vi "对非本VI中控件属性操作.vi"() -> ()   [LabVIEW 2018]
uses:
  <vilib>/Utility/error.llb/DialogType.ctl
  <vilib>/Utility/miscctls.llb/LVPointTypeDef.ctl
  <vilib>/Utility/file.llb/Read Delimited Spreadsheet (string).vi
  <vilib>/Utility/file.llb/Write Delimited Spreadsheet (string).vi
panel:
  in  "下拉列表":T1 items=["Digital"]
  in  "界面控件":T2 {"下拉列表" items=["Digital"]}
  in  "选项卡控件":enum32{"基本设置", "控件外观设置", "创建控件"}(tab)
  in  "获取控件名称":bool
  in  "重定原点":bool
  in  "获取控件引用":bool
  in  "流量控件设置":bool
  in  "电流控件设置":bool
  in  "温度控件设置":bool
  in  "压力压差控件设置":bool
  in  "创建数量":u16
  in  "创建T控件":bool
  in  "停止":bool
  out "Error Report":string
  out "Dynamic Threads Array":string[](array[string])
  out "Current State":string
  in  "OK":bool
  in  "Exit Program":bool
  in  "Load Dynamic VI":bool
  in  "Close Dynamic VI":bool
  in  "Load Engine VI":bool
  in  "Close Engine VI":bool
  in  "Load Reentrant VI":bool
  out "数值":i32
  in  "颜色盒 2":u32(colorbox)
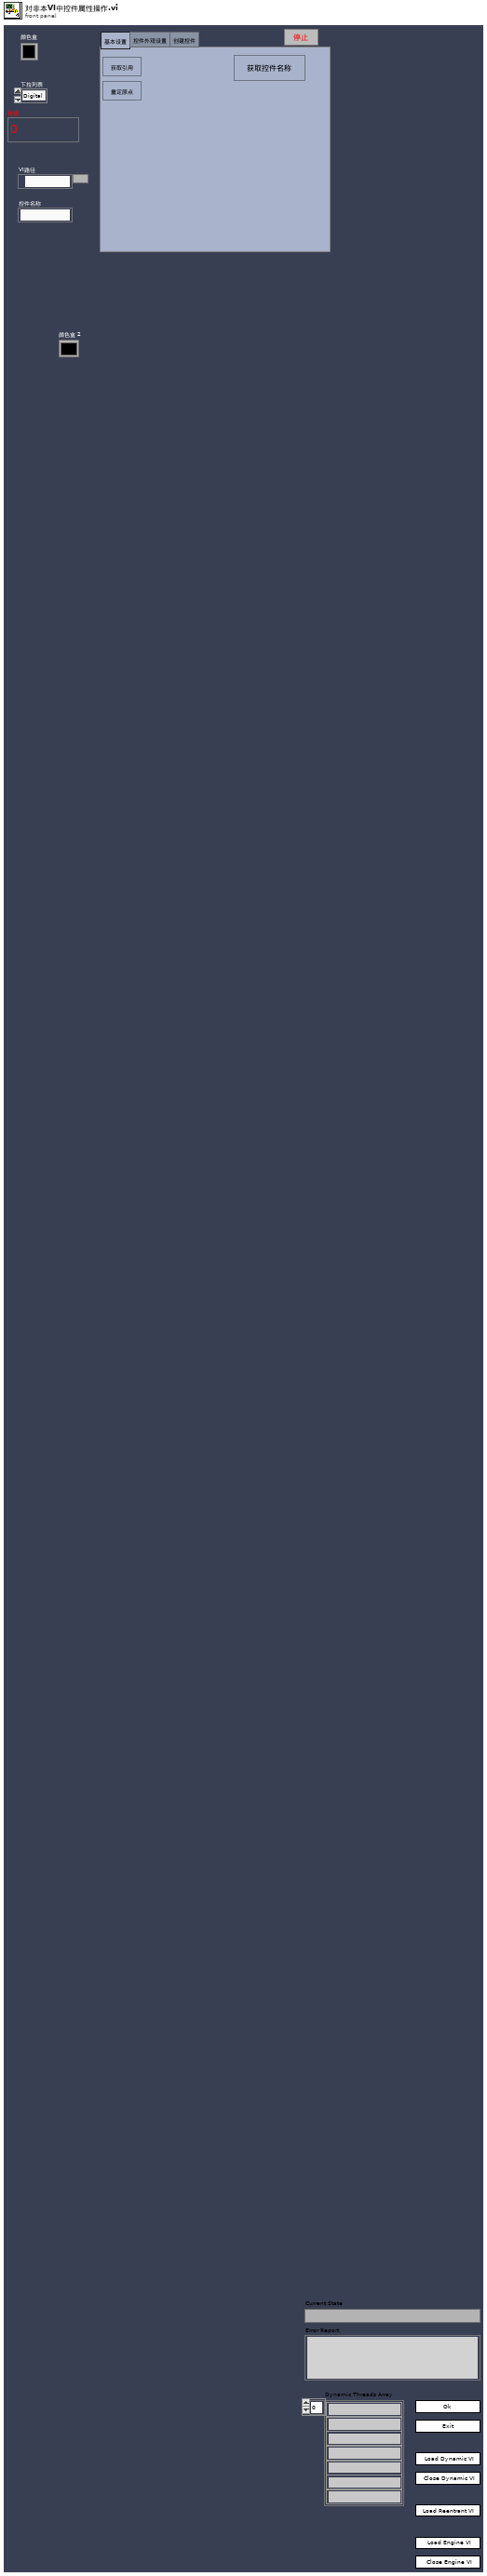
[diagram p1: front panel]
types:
  T1 = typedef "类名.ctl" = u16
  T2 = cluster{"颜色盒":u32, "下拉列表":T1, "VI路径":path, "控件名称":string}
  T3 = typedef "LVPointTypeDef.ctl" = cluster{"Horizontal":i16, "Vertical":i16}
  T4 = typedef "LVBoundsTypeDef.ctl" = cluster{"Width":u32, "Height":u32}
  T5 = typedef "LVFontTypeDef.ctl" = cluster{"Font Name":string, "Size":u16, "Bold":bool, "Italic":bool, "Underline":bool, "Strikeout":bool, "Color":u32}
  T6 = typedef "DynamicThreads.ctl" = cluster{"ReOriginVI":path}
  T7 = cluster{"Error":errorcluster, "Exit":bool, "All Ref":cluster{"VIRef":refnum<vi>, "CtlRef":refnum<vi>, "界面控件Ref":refnum<vi>}, "System Path":cluster{"Data":path}, "Dynamic VI Path":cluster{"Thread Path":path}, "Reentrant VI Path":cluster{"Reentrant Thread Path":path, "Reentrant VI Count":u32}, "Engine Path":cluster{"Engine Path":path}, "Main VI":cluster{"Main Name":string, "Main Order":string, "Main Data":variant}, "Engine":cluster{"Engine Path":path, "Engine Name":string, "Engine Order":string, "Engine Data":variant}, "Thread to Operate":cluster{"Thread VI Path":path, "Invoke Property":cluster{"open front panel? (T)":bool, "Reentrant? (F)":bool, "Insert to Subpanel?(F)":bool, "time out(5s)":dbl}, "Queue Info":cluster{"HighLevel Thread":string, "Thread Q Name":string, "Data":variant}}, "Send Data to Thread":cluster{"Thread to Send":string[], "Order to Send":string[], "Data to Send":variant[]}, "Dynamic Threads Array":string[], "控件排布前面板":cluster{"获取引用":cluster{"获取VI引用句柄":refnum<vi>, "获取Ctl引用句柄":refnum<vi>}, "位置_前":cluster{"位置":T3}, "创建控件":cluster{"创建数量":u16}, "lNameLable":string[]}, "控件排布后面板":cluster{"位置_后":cluster{"位置":T3}}, "DynamicThreadsPath":T6, "界面控件":cluster{"当前选择路径":path, "控件名称":string, "颜色盒":u32, "名称列表路径":path, "名称列表":string[], "类名":string}}
  T8 = enum32{"Invalid", "Standard", "Closed", "Hidden", "Minimized", "Maximized"}
  T9 = cluster{"open front panel? (T)":bool, "Reentrant? (F)":bool, "Insert to Subpanel?(F)":bool, "time out(5s)":dbl}
  T10 = typedef "DialogType.ctl" = u16
  T11 = cluster{"HighLevel Thread":string, "Thread Q Name":string, "Data":variant}
  T12 = cluster{"颜色盒":bool, "下拉列表":bool, "VI路径":bool, "控件名称":bool}
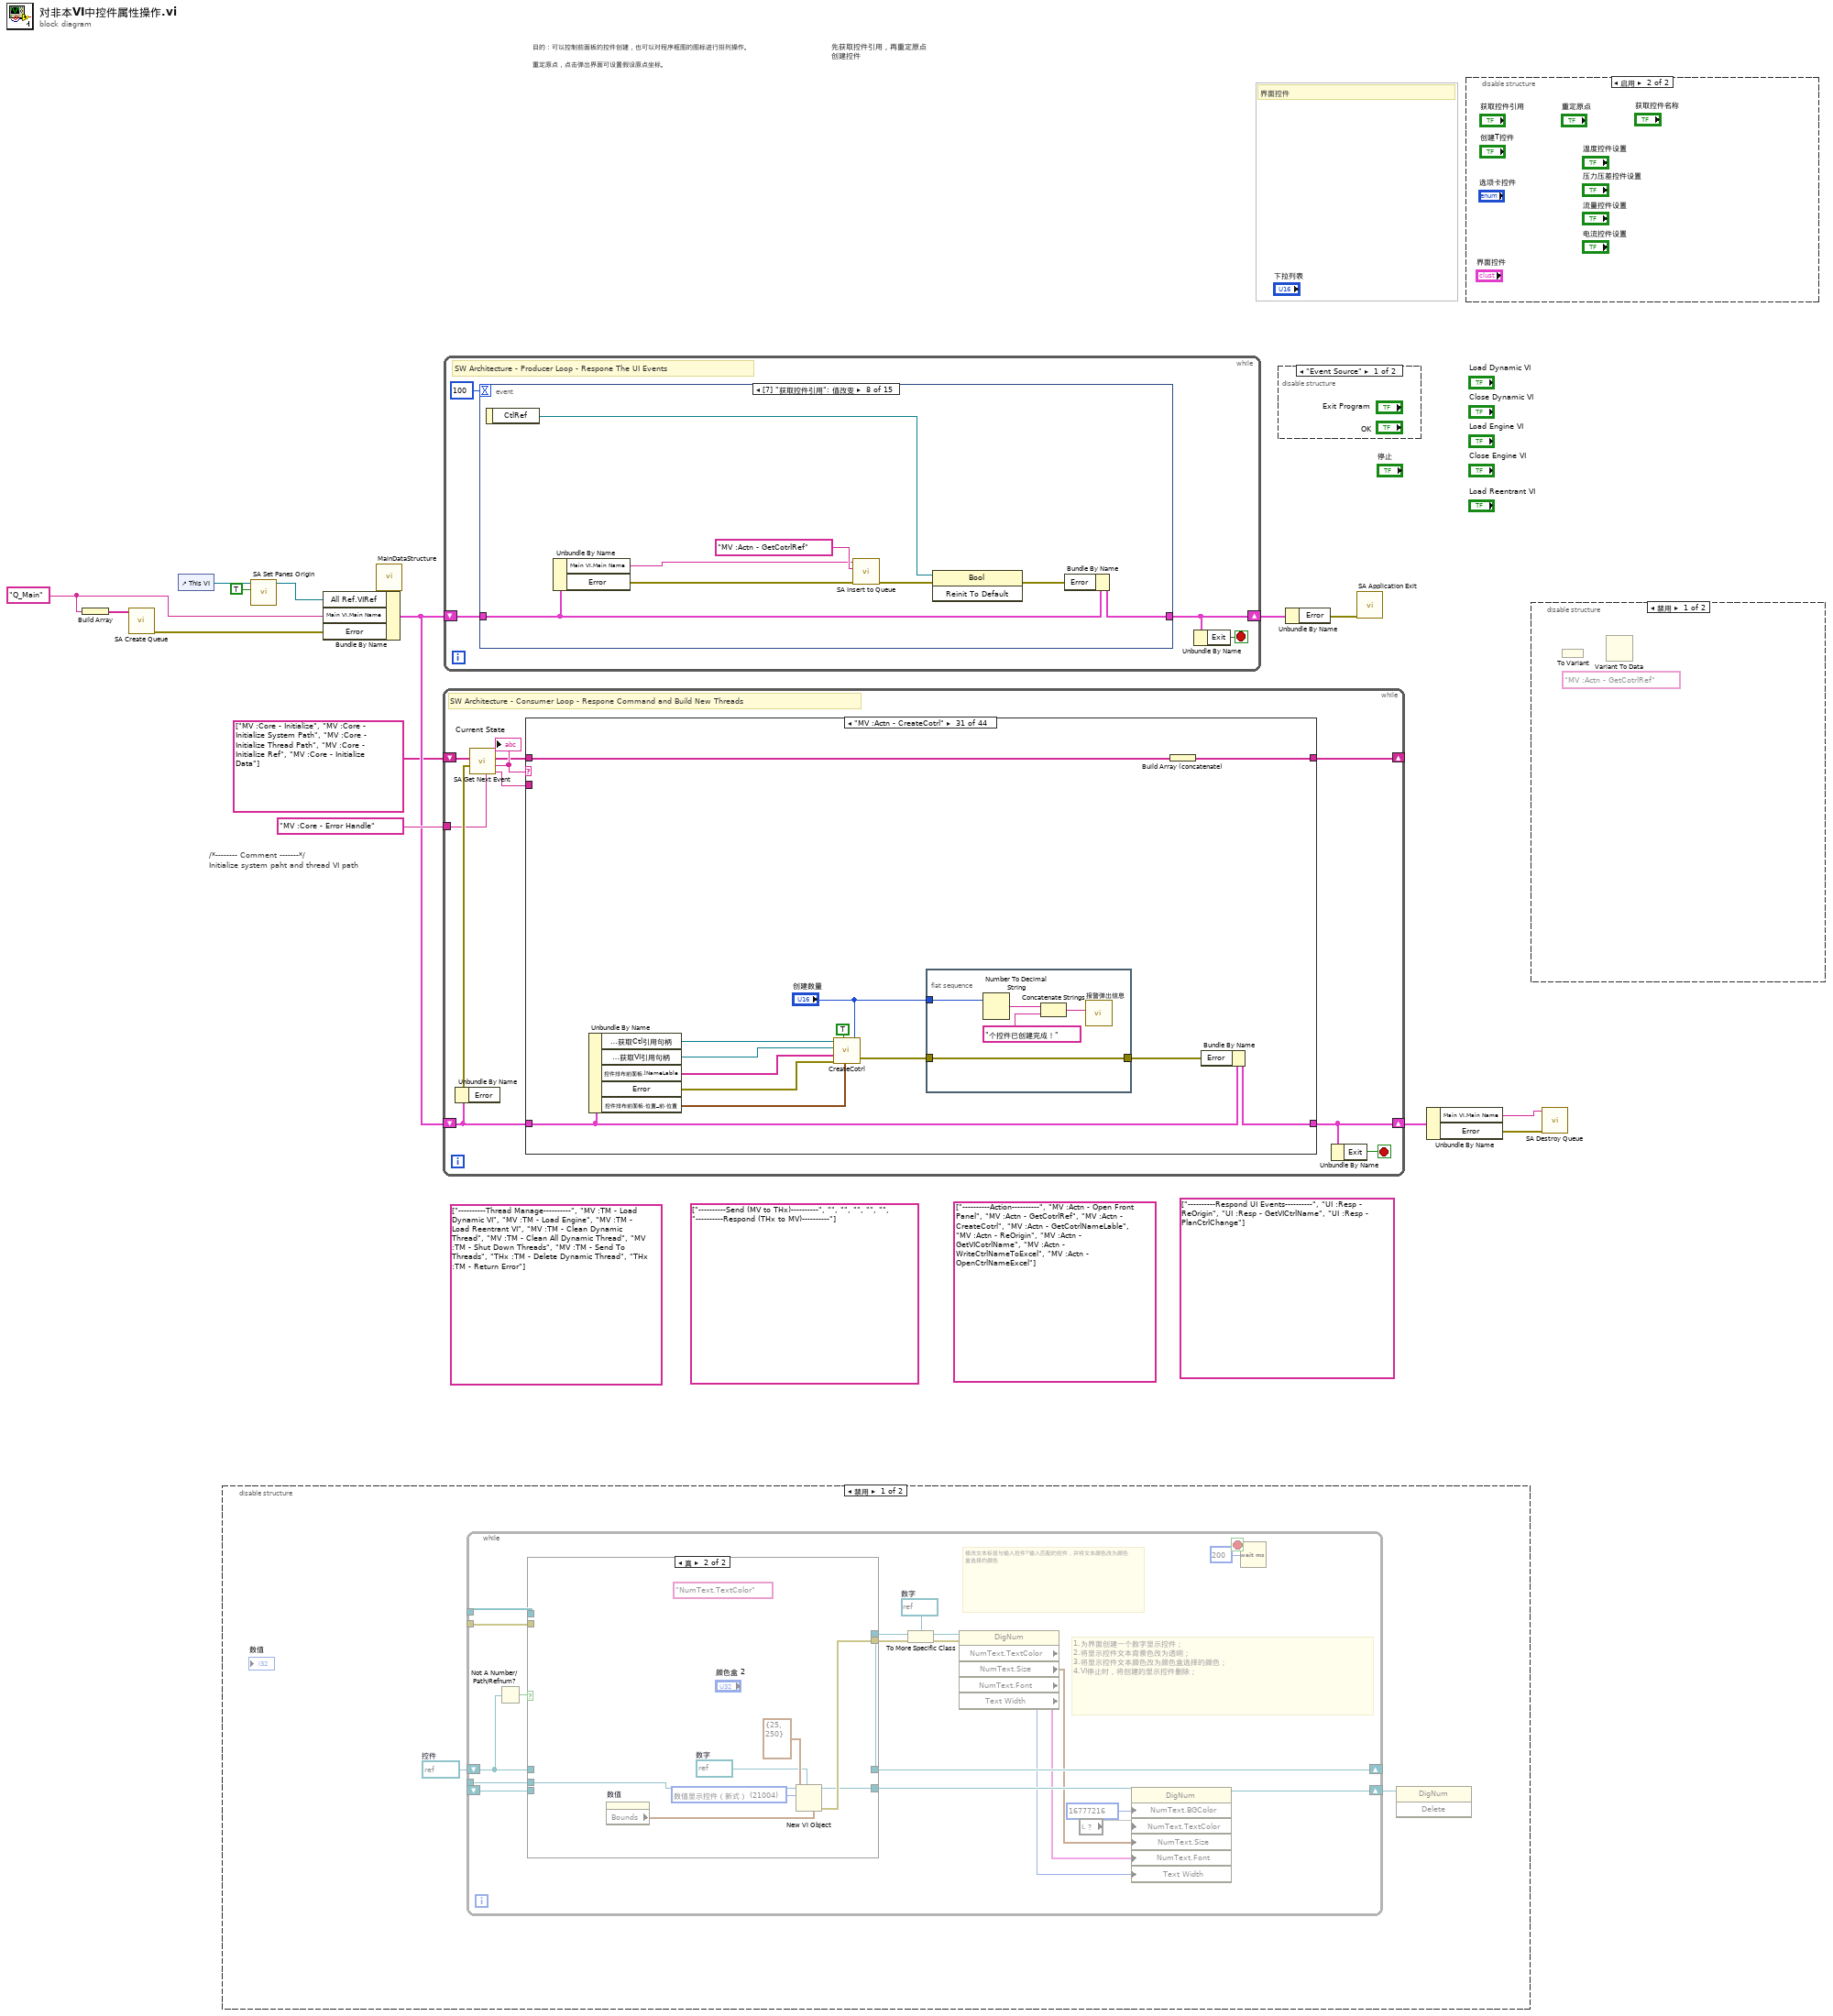
[diagram p0: block diagram]
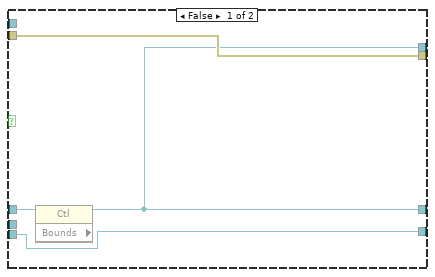
[diagram p4: hidden frame]
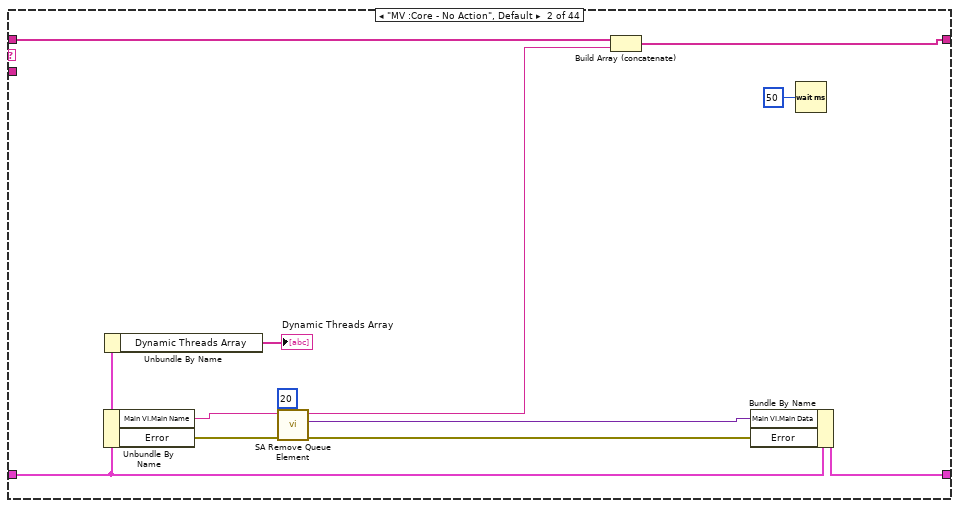
[diagram p8: hidden frame]
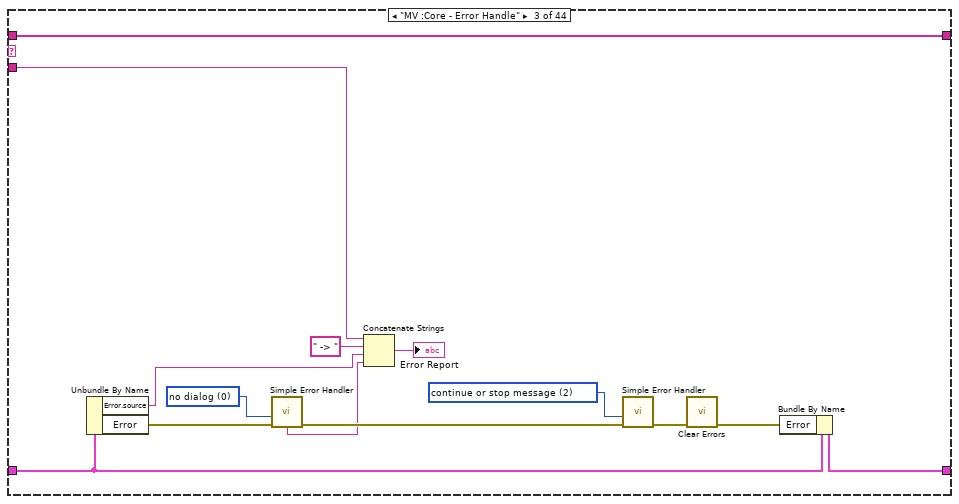
[diagram p9: hidden frame]
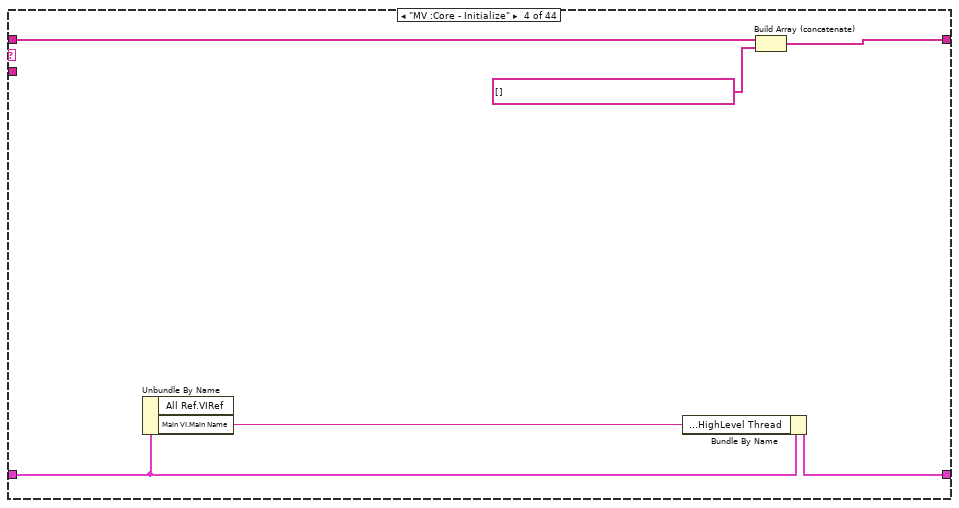
[diagram p10: hidden frame]
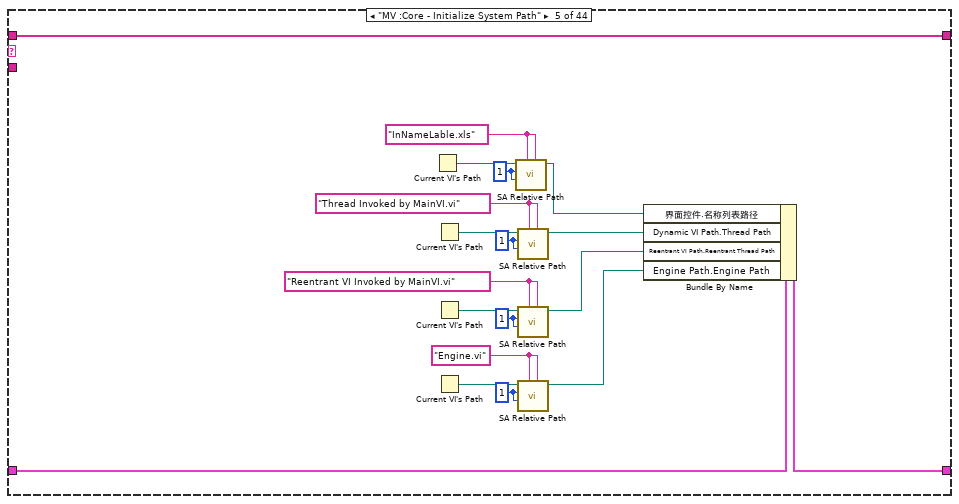
[diagram p11: hidden frame]
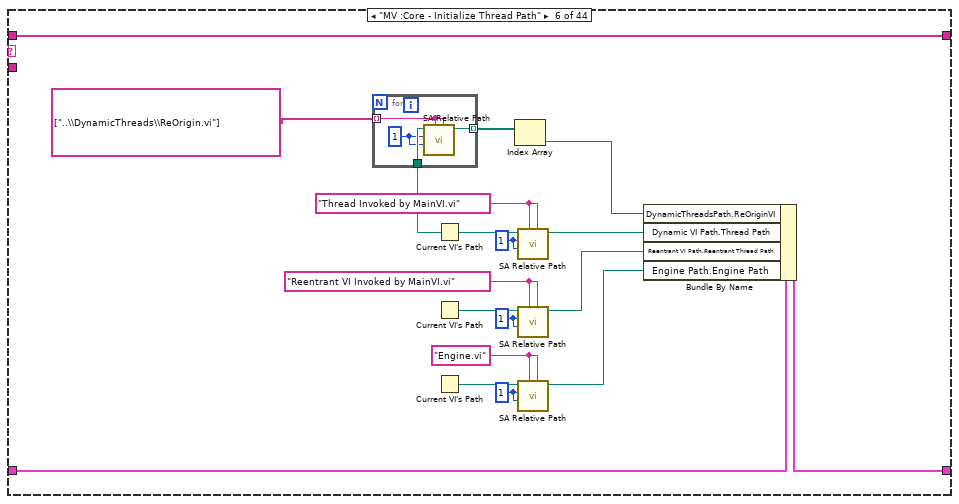
[diagram p12: hidden frame]
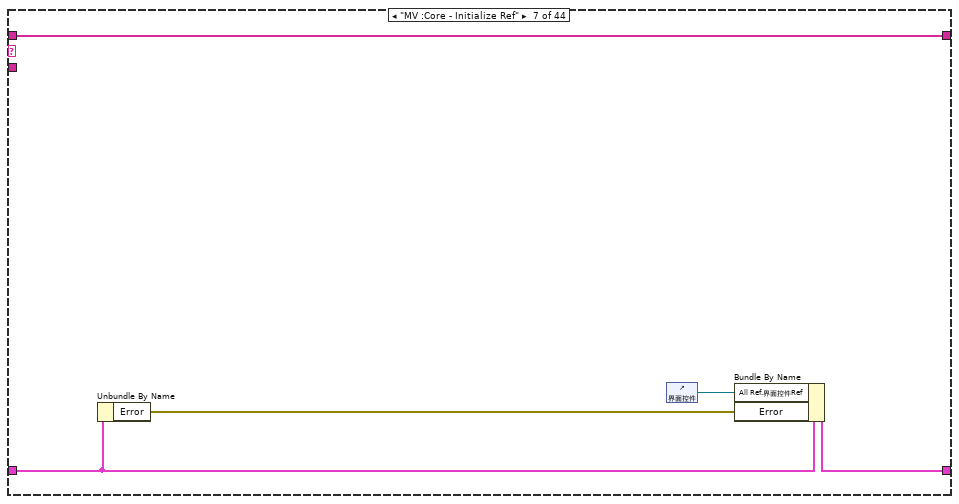
[diagram p13: hidden frame]
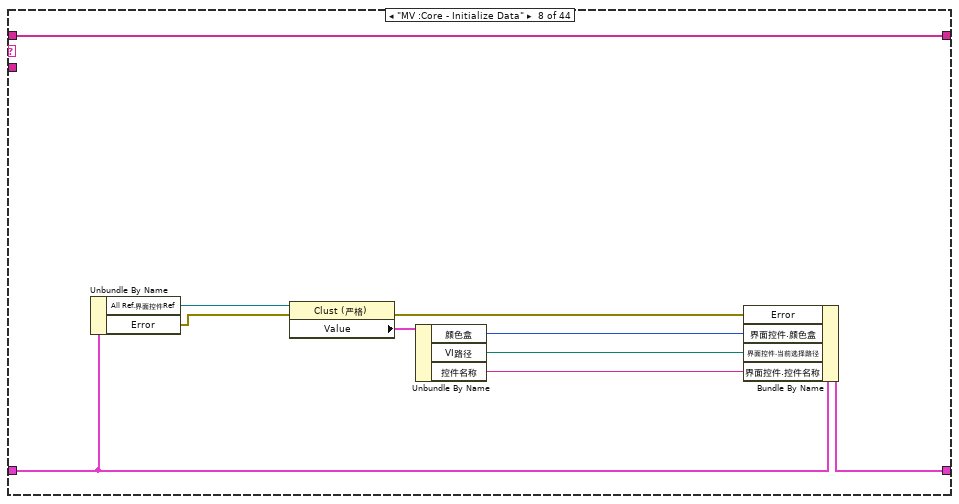
[diagram p14: hidden frame]
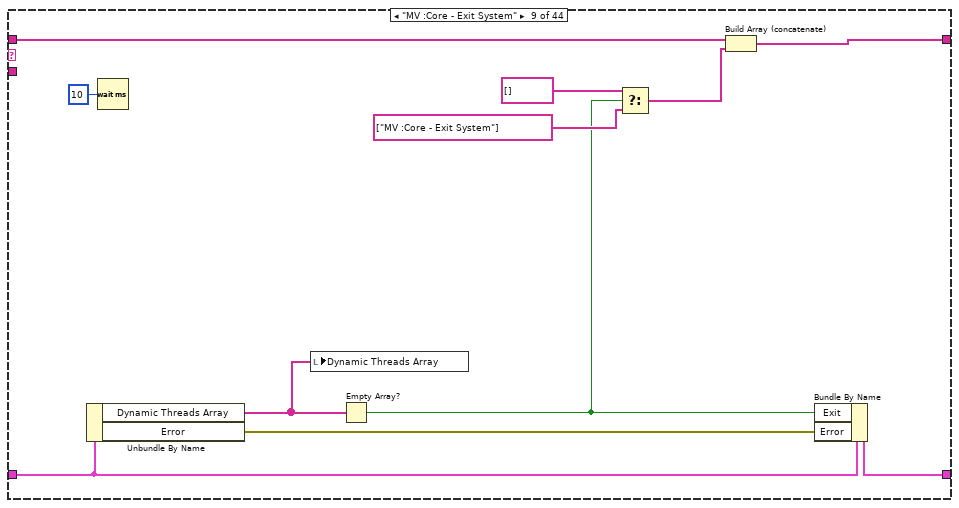
[diagram p15: hidden frame]
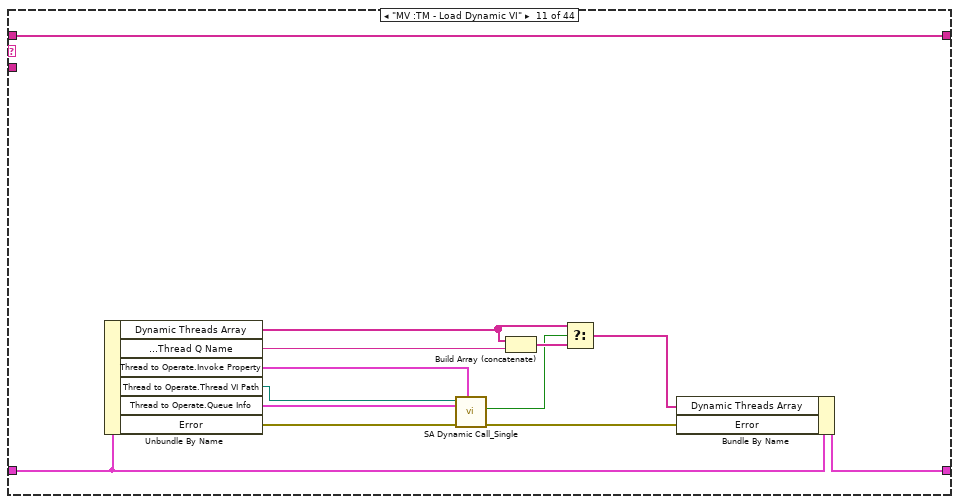
[diagram p17: hidden frame]
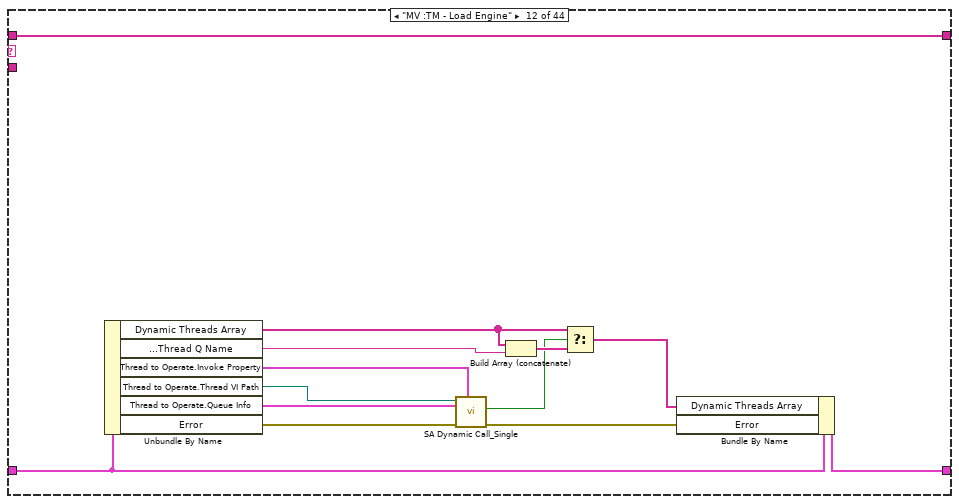
[diagram p18: hidden frame]
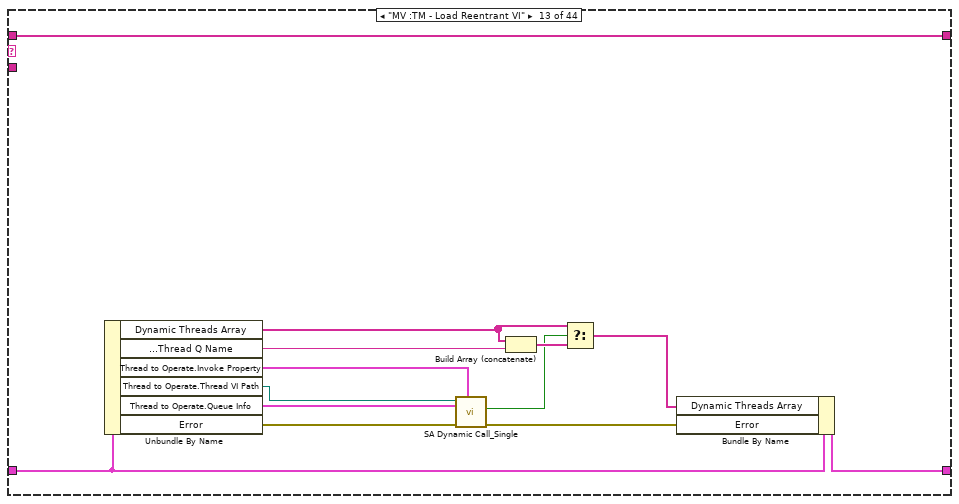
[diagram p19: hidden frame]
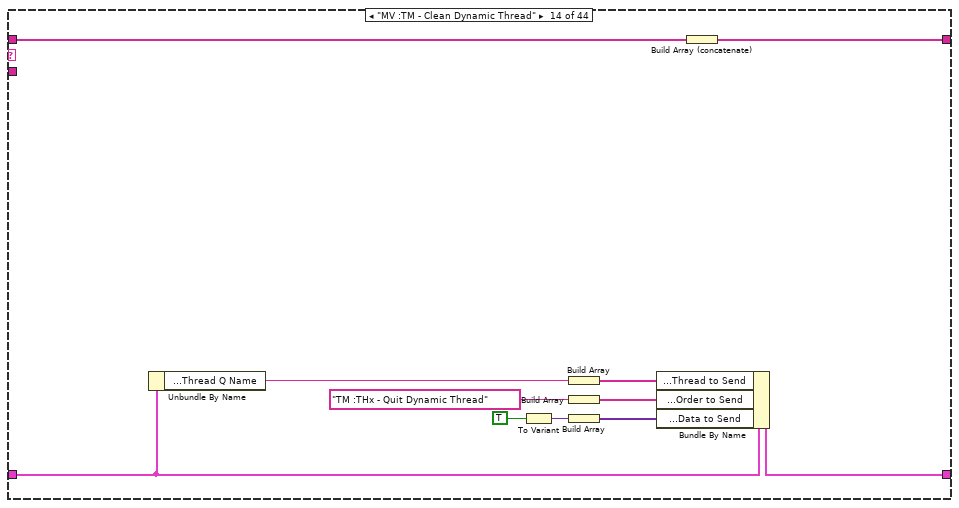
[diagram p20: hidden frame]
diagram:
  (unwired) string[] ["----------Action----------", "MV :Actn - Open Front Panel", "MV :Actn - GetCotrlRef", "MV :Actn - CreateCotrl", "MV :Actn - GetCotrlNameLable", "MV :Actn - ReOrigin", "MV :Actn - GetVICotrlName", "MV :Actn - WriteCtrlNameToExcel", "MV :Actn - OpenCtrlNameExcel"]
  (unwired) string[] ["----------Respond UI Events----------", "UI :Resp - ReOrigin", "UI :Resp - GetVICtrlName", "UI :Resp - PlanCtrlChange"]
  (unwired) string[] ["----------Send (MV to THx)----------", "", "", "", "", "", "----------Respond (THx to MV)----------"]
  (unwired) string[] ["----------Thread Manage----------", "MV :TM - Load Dynamic VI", "MV :TM - Load Engine", "MV :TM - Load Reentrant VI", "MV :TM - Clean Dynamic Thread", "MV :TM - Clean All Dynamic Thread", "MV :TM - Shut Down Threads", "MV :TM - Send To Threads", "THx :TM - Delete Dynamic Thread", "THx :TM - Return Error"]
  w9 = "Q_Main" ("Queue name(unamed)")
  # "界面控件"
  # "目的：可以控制前面板的控件创建，也可以对程序框图的图标进行排列操作。\n\n重定原点，点击弹出界面可设置假设原点坐标。"
  # "先获取控件引用，再重定原点\n创建控件"
  # "/*-------- Comment -------*/\nInitialize system paht and thread VI path"
  n1 = Build Array(w9) -> (w10:string[])
  n2 = call <vilib>:"SA Create Queue.vi"("Queue Name"=w10) -> ("error out"=w6:errorcluster)  [unwired: 10 in]
  n3 = control-ref of="This VI"() -> (w13:refnum<vi>)
  n4 = disable-structure shown="禁用" {
    frame Disabled {
      w18 = refnum<vi> refnum  # 控件
      n5 = while {
        tunnel: _ -> [w38]
        tunnel: _ -> [w39]
        shift-right: [w31] -> _
        shift-left: w18 -> [w29]
        tunnel: [w27] -> w16
        shift-right: [w24] -> w17
        shift-left: _ -> [w22]
        stop <- _ stop-if-true
        w36 = refnum<vi> refnum  # 数字
        # "修改文本标签与输入控件Y输入匹配的控件，并将文本颜色改为颜色盒选择的颜色"
        # "1.为界面创建一个数字显示控件；\n2.将显示控件文本背景色改为透明；\n3.将显示控件文本颜色改为颜色盒选择的颜色；\n4.VI停止时，将创建的显示控件删除；"
        n6 = Not A Number/Path/Refnum?(number/path/refnum=w29) -> (NaN/Path/Refnum?=w30:bool)
        n7 = case shown="真" w30 {
          tunnel: w39 -> [w43 _]
          tunnel: w38 -> [_ _]
          tunnel: [w43 w48] -> w33
          tunnel: [w41 w47] -> w28
          tunnel: [w41 w47] -> w31
          tunnel: w29 -> [w42 _]
          tunnel: w27 -> [_ w46]
          tunnel: [w40 w45] -> w23
          tunnel: w22 -> [w40 _]
          frame False {
            n8 = property class="Ctl" props=["Bounds"](reference=w42) -> (reference out=w41:refnum<vi>)  [unwired: 1 in, 2 out]
          }
          frame True {
            w49 = refnum<vi> refnum  # 数字
            w51 = 21004 items=[".NET容器"=2125, ".NET引用句柄"=3441, "10的幂"=1212, "10的自然对数"=23513, "2的幂"=1223, "2的自然对数"=23514, "ActiveX容器"=2072, "Agitator"=3831, "Array Interface Control"=23777, "Bin#1"=3073, "Bin#2"=21755, "CAN接口（程序框图常量）"=2123, "CAN接口（经典）"=3339, "CAN接口（系统）"=21964, "CAN接口（新式）"=21815, "CAN任务（程序框图常量）"=3471, "CAN任务（经典）"=3470, "CAN任务（系统）"=21963, "CAN任务（新式）"=21789, "CAN通道（程序框图常量）"=2124, "CAN通道（经典）"=3340, "CAN通道（系统）"=21966, "CAN通道（新式）"=21817, "CPU信息"=24130, "DAQmx换算名（程序框图常量）"=2116, "DAQmx换算名（经典）"=3317, "DAQmx换算名（系统）"=21952, "DAQmx换算名（新式）"=21775, "DAQmx接线端（程序框图常量）"=2117, "DAQmx接线端（经典）"=3319, "DAQmx接线端（系统）"=21955, "DAQmx接线端（新式）"=21781, "DAQmx开关（程序框图常量）"=2121, "DAQmx开关（经典）"=3337, "DAQmx开关（系统）"=21953, "DAQmx开关（新式）"=21776, "DAQmx模拟触发器源（程序框图常量）"=2119, "DAQmx模拟触发器源（经典）"=3336, "DAQmx模拟触发器源（系统）"=21951, "DAQmx模拟触发器源（新式）"=21774, "DAQmx全局通道（程序框图常量）"=3430, "DAQmx全局通道（经典）"=3443, "DAQmx全局通道（系统）"=21957, "DAQmx全局通道（新式）"=21770, "DAQmx任务名（程序框图常量）"=3434, "DAQmx任务名（经典）"=3442, "DAQmx任务名（系统）"=21959, "DAQmx任务名（新式）"=21778, "DAQmx设备名（程序框图常量）"=2093, "DAQmx设备名（经典）"=3318, "DAQmx设备名（系统）"=21950, "DAQmx设备名（新式）"=21773, "DAQmx物理通道（程序框图常量）"=2118, "DAQmx物理通道（经典）"=3335, "DAQmx物理通道（系统）"=21954, "DAQmx物理通道（新式）"=21777, "DataSocket引用句柄"=3417, "EOF"=1410, "exp(x)-1"=1222, "e的倒数"=23511, "FieldPoint IO点（程序框图常量）"=3440, "FieldPoint IO点（经典）"=3439, "FieldPoint IO点（新式）"=21784, "FIFO引用句柄"=3474, "For循环"=2002, "FPGA引用句柄至会话句柄转换"=2322, "Furnace"=3829, "GPIB初始化"=1957, "GPIB触发"=1953, "GPIB串行轮询"=1955, "GPIB等待"=1958, "GPIB读取"=1951, "GPIB其他命令"=1956, "GPIB清零"=1954, "GPIB写入"=1950, "GPIB状态"=1959, "IMAQ会话句柄"=3415, "IP地址至字符串转换"=1710, "IVI逻辑名称（程序框图常量）"=3420, "IVI逻辑名称（经典）"=3414, "IVI逻辑名称（新式）"=21736, "IVI删除会话句柄"=8103, "IVI新建会话句柄"=8102, "LabVIEW对象"=3457, "Mac对话组合框"=32514, "MathScript节点"=2357, "MATLAB脚本"=9020, "OLE变体"=3150, "Pi"=23504, "Pi乘以2"=23505, "Pi除以2"=23506, "Pi的倒数"=23507, "Pi的自然对数"=23508, "Python会话引用句柄"=3486, "Python节点"=24205, "RT FIFO创建"=24000, "RT FIFO读取"=24001, "RT FIFO删除"=24003, "RT FIFO写入"=24002, "Simon量表"=32600, "Sinc"=1227, "TCP平化读取"=1718, "TCP平化写入"=1719, "TCP网络连接引用句柄"=3407, "TCP自由读取"=1720, "TCP自由写入"=1721, "TDMS Close"=24113, "TDMS Defragment"=24119, "TDMS Flush"=24117, "TDMS Get Properties"=24115, "TDMS List Contents"=24116, "TDMS Open"=24112, "TDMS Read"=24111, "TDMS Refnum To File ID"=24120, "TDMS Set Properties"=24114, "TDMS Write"=24110, "TDMS Write IP"=24118, "TDMS获取异步读取状态（数据引用）"=2155, "TDMS获取异步写入状态（数据引用）"=2154, "TDMS内存中打开"=2156, "TDMS内存中读取字节"=2158, "TDMS内存中关闭"=2157, "TDMS配置异步读取（数据引用）"=2153, "TDMS配置异步写入（数据引用）"=2152, "TDMS删除数据"=2159, "TDMS文件"=3477, "UDP网络连接引用句柄"=3418, "UTF-8至文本转换"=23067, "VISA GPIB传递IFC"=2318, "VISA GPIB传递控制权"=2317, "VISA GPIB控制ATN"=2316, "VISA GPIB控制REN"=2304, "VISA GPIB命令"=2315, "VISA USB控制输出"=2087, "VISA USB控制输入"=2086, "VISA VXI命令或查询"=2305, "VISA查找资源"=1923, "VISA存数16"=1935, "VISA存数32"=1996, "VISA存数64"=2143, "VISA存数8"=1939, "VISA打开"=2308, "VISA等待事件"=1943, "VISA读取"=1925, "VISA读取STB"=1928, "VISA读取设备并写入文件"=2313, "VISA读取文件并写入设备"=2314, "VISA放弃事件"=1941, "VISA关闭"=1922, "VISA解锁"=1994, "VISA禁用事件"=1940, "VISA内存分配"=1997, "VISA内存分配Ex"=2146, "VISA内存释放"=1998, "VISA启用事件"=1942, "VISA清空I/O缓冲区"=2302, "VISA取数16"=1934, "VISA取数32"=1995, "VISA取数64"=2142, "VISA取数8"=1938, "VISA取消触发映射"=2312, "VISA取消地址映射"=1933, "VISA设备清零"=1927, "VISA设置I/O缓冲区大小"=2301, "VISA输出16"=1931, "VISA输出32"=1945, "VISA输出64"=2141, "VISA输出8"=1937, "VISA输入16"=1930, "VISA输入32"=1944, "VISA输入64"=2140, "VISA输入8"=1936, "VISA锁"=1993, "VISA写入"=1926, "VISA引用句柄至会话句柄转换"=2300, "VISA映射触发"=2311, "VISA映射地址"=1932, "VISA置触发有效"=1929, "VISA置效用信号有效"=2310, "VISA置中断信号有效"=2309, "VISA转出16"=1949, "VISA转出32"=1992, "VISA转出64"=2145, "VISA转出8"=1947, "VISA转入16"=1948, "VISA转入32"=1991, "VISA转入64"=2144, "VISA转入8"=1946, "VISA转移"=2303, "VISA状态说明"=1924, "VISA资源名称"=3421, "VISA资源名称（经典）"=3409, "VISA资源名称（新式）"=21737, "VI服务器引用"=2091, "VI库"=1425, "VI引用句柄"=3422, "While循环#1"=2003, "While循环#2"=2352, "XY图（经典）"=3500, "XY图（新式）"=21716, "X的Y次根"=23062, "X的幂"=1213, "阿伏加德罗常数(1/mol)"=23520, "按2的幂缩放"=1074, "按名称解除捆绑"=2058, "按名称捆绑"=2057, "按索引获取控件值"=24204, "按索引设置控件值"=24203, "八进制数？"=1129, "八进制字符串至数值转换"=1186, "包矩阵"=23001, "包括定点溢出状态"=5564, "保留运行类"=8018, "比特包至数组"=3135, "闭包结构"=2372, "变量类说明符常量"=2106, "变量名称常量"=3478, "变体"=3310, "变体至平化字符串转换"=8203, "变体至数据转换"=8003, "标签（系统）"=21961, "标签（新式）"=21960, "标识符属性下拉列表"=2063, "表达式节点"=2201, "表格（经典）"=21796, "表格（系统）"=21797, "表格（新式）"=21790, "并行轮询"=1969, "并行轮询配置"=1970, "波形图（经典）"=3504, "波形图（新式）"=21703, "波形图表"=21010, "波形图表（经典）"=3501, "波形图表（新式）"=21717, "不等于0？"=1116, "不等于？"=1105, "布尔数组至数值转换"=1815, "布尔值至(0,1)转换"=1167, "步进数值控件（系统）"=21900, "彩色矩形（断开？）"=3625, "菜单下拉列表（经典）"=3018, "菜单下拉列表（新式）"=21600, "菜单引用句柄"=3413, "测试SRQ"=1986, "层叠式顺序结构"=2000, "插入菜单项"=9003, "插入式控件"=21820, "查找请求设备"=1966, "查找通道探针"=9155, "查找侦听器"=1965, "拆分按钮"=21020, "拆分路径"=1420, "拆分数字"=1170, "拆分信号"=2351, "拆分一维数组"=1908, "产生前面板活动"=1329, "产生事件发生"=1700, "产生用户定义Trace事件"=2250, "产生用户事件"=2074, "敞口槽（经典）"=3070, "敞口槽（新式）"=21751, "敞口罐（平面，经典）"=21752, "敞口罐（阴影，经典）"=3074, "乘"=1052, "乘（带错误接线端）"=3917, "程序框图禁用结构"=2054, "抽取一维数组"=2046, "初始化数组"=2053, "除"=1053, "除（带错误接线端）"=3918, "触发"=1988, "触发设备列表"=1989, "传递控制权"=1968, "传送器"=3827, "传统DAQ通道（程序框图常量）"=2085, "传统DAQ通道（经典）"=3320, "传统DAQ通道（新式）"=21733, "串行轮询所有设备"=1960, "创建TCP侦听器"=1717, "创建波形"=2066, "创建簇数组"=2047, "创建红外线侦听器"=9140, "创建矩阵"=8500, "创建蓝牙侦听器"=9151, "创建流"=23796, "创建路径"=1419, "创建数组"=2041, "创建网络流读取方端点"=23811, "创建网络流端点"=23793, "创建网络流写入方端点"=23810, "创建唯一网络流读取方端点"=23807, "创建唯一网络流端点"=23795, "创建唯一网络流写入方端点"=23806, "创建文件夹"=8055, "创建用户事件"=2073, "垂直分隔栏"=21860, "垂直分隔栏（经典）"=21862, "垂直分隔栏（系统）"=21864, "垂直管道（平面）"=3816, "垂直管道（阴影）"=3716, "垂直滚动条"=21111, "垂直滑动杆（系统）"=21903, "垂直滑动杆开关（经典）"=3115, "垂直滑动杆开关（新式）"=21741, "垂直进度条（系统）"=21909, "垂直进度条（新式）"=21104, "垂直开关"=3109, "垂直刻度条"=21107, "垂直平滑盒"=3634, "垂直翘板开关"=21740, "垂直梯度矩形"=32503, "垂直梯度椭圆"=32501, "垂直梯度圆角矩形"=32506, "垂直填充滑动杆（经典）"=3009, "垂直填充滑动杆（新式）"=21014, "垂直摇杆开关（经典）"=3111, "垂直摇杆开关（新式）"=21005, "垂直直线"=3822, "垂直指针滑动杆（经典）"=3007, "垂直指针滑动杆（系统）"=21901, "垂直指针滑动杆（新式）"=21017, "从JSON还原"=24202, "从XML还原"=8401, "从流中读取单个元素"=23797, "从流中读取多个元素"=23803, "从之前设备中读取数据"=1972, "从字符串还原"=1165, "簇（经典）"=3400, "簇（新式）"=21607, "簇常量"=2071, "簇至数组转换"=1169, "错误下拉列表常量"=2039, "打开/创建/替换数据记录文件"=8054, "打开/创建/替换文件"=8050, "打开DataSocket"=1084, "打开Python会话"=24206, "打开TCP连接"=1715, "打开UDP"=1723, "打开UDP多点传送"=1727, "打开VI对象引用"=8013, "打开VI引用"=8010, "打开变量连接"=23779, "打开并验证变量连接"=23790, "打开动态比特文件引用"=5691, "打开红外线连接"=9142, "打开蓝牙连接"=9153, "打开设备"=1430, "打开文件"=1403, "打开应用程序引用"=8012, "打开自动化"=8000, "大于0？"=1117, "大于？"=1110, "大于等于0？"=1114, "大于等于？"=1103, "带边框颜色盒（经典）"=3008, "带边框颜色盒（新式）"=21019, "带标签方形按钮"=3123, "带标签矩形按钮"=3124, "带标签椭圆形按钮"=3125, "带标签圆形按钮"=3122, "带箭头线（粗）"=3631, "带箭头线（细）"=3628, "带进位的右移位"=1607, "带进位的左移位"=1606, "带阴影的椭圆"=32509, "带阴影的圆角矩形"=32508, "代码接口节点"=2050, "单按钮对话框"=1340, "单位转换"=2059, "单选按钮（经典）"=22003, "单选按钮（系统）"=3133, "单选按钮（系统） 1"=22002, "单选按钮（新式）"=22001, "弹出菜单下拉列表"=3017, "当前VI菜单栏"=9000, "当前VI路径"=1426, "当前进程ID"=24131, "倒数"=1059, "等待(ms)"=1302, "等待GPIB RQS"=1952, "等待SRQ"=1990, "等待TCP侦听器"=1712, "等待带通知器历史的多个通知"=9132, "等待带通知器历史的通知"=9131, "等待多个通知"=9106, "等待红外线侦听器"=9143, "等待活动"=1722, "等待蓝牙侦听器"=9147, "等待前面板活动"=1328, "等待事件发生"=1701, "等待通知"=9105, "等待下一个整数倍毫秒"=1327, "等于0？"=1113, "等于？"=1102, "底数为10的对数"=1210, "底数为2的对数"=1225, "底数为X的对数"=1224, "电子表格字符串至数组转换"=1539, "调用父方法"=2354, "调用节点"=3900, "调用库函数节点"=2062, "调用链"=1999, "调整矩阵大小"=8508, "定点溢出？"=5565, "定点转换为整型"=5566, "定时顺序"=5573, "定时循环"=5570, "动态FPGA接口转换"=5690, "读取DataSocket"=1086, "读取TCP数据"=1716, "读取UDP数据"=1724, "读取变量"=23781, "读取变量（超时方式）"=23786, "读取二进制文件"=8051, "读取红外线数据"=9145, "读取蓝牙数据"=9149, "读取设备"=1432, "读取数据记录文件"=8069, "读取文本文件"=8070, "读取文件"=1407, "读取状态"=1973, "队列引用句柄"=3424, "队列最前端插入元素"=9129, "对话框垂直滚动条"=21906, "对话框数值#1"=2100, "对话框数值#2"=3006, "对话框水平滚动条"=21905, "对话框字符串"=2110, "多段管道"=23780, "多列列表框（经典）"=21799, "多列列表框（系统）"=21798, "多列列表框（新式）"=21791, "多速率结构"=2199, "二维数组转置"=1902, "二维图片"=3508, "发动机（平面）"=3820, "发动机（阴影）"=3720, "发送"=1977, "发送IFC"=1980, "发送LLO"=1982, "发送命令"=1978, "发送设置"=1983, "发送数据"=1979, "发送通知"=9104, "发送至设备列表"=1981, "反馈节点"=2353, "反双曲余割"=23056, "反双曲余切"=23058, "反双曲余弦"=1218, "反双曲正割"=23057, "反双曲正切"=1219, "反双曲正弦"=1217, "反余割"=23050, "反余切"=23052, "反余弦"=1207, "反正割"=23051, "反正切"=1208, "反正切（2个输入）"=1228, "反正弦"=1206, "反转一维数组"=1900, "反转字符串"=1537, "方形按钮"=3101, "方形单选按钮"=3107, "方形灯"=3105, "方形开关按钮"=3119, "方形开关按钮（性能分析）"=3113, "方形指示灯（经典）"=3121, "方形指示灯（新式）"=21013, "访问权限"=1412, "非"=1064, "非法共享变量"=23527, "非法路径常量"=23524, "非法数字/路径/引用句柄？"=1128, "非法引用句柄常量"=23526, "分叉"=2194, "分解变体"=2404, "分解锁定数据变量引用"=2406, "分数/指数字符串至数值转换"=1187, "符号"=1049, "浮点数等于？"=23064, "复共轭"=1048, "复合运算"=2200, "复数至极坐标转换"=1045, "复数至实部虚部转换"=1044, "复选框（经典）"=3117, "复选框（系统）"=3132, "复选框（新式）"=21924, "复制"=8053, "复制（过时）"=1416, "负无穷大"=23509, "高级TDMS异步读取（数据引用）"=2151, "高级TDMS异步写入（数据引用）"=2150, "格式化日期/时间字符串"=8100, "格式化写入文件"=2083, "格式化写入字符串"=2081, "格式化值"=1512, "公式节点"=2004, "共享变量"=23778, "共享变量常量"=3473, "共享变量控件（经典）"=3472, "共享变量控件（新式）"=21814, "共享变量至字符串转换"=1831, "构造器节点"=3904, "关闭DataSocket"=1085, "关闭Python会话"=24207, "关闭TCP连接"=1713, "关闭UDP"=1726, "关闭变量连接"=23783, "关闭红外线连接"=9144, "关闭蓝牙连接"=9148, "关闭文件"=8052, "关闭文件（已停用 ）"=1405, "关闭引用"=8011, "关闭自动化"=8001, "合并错误"=2147, "合并信号"=2350, "红外线网络连接引用句柄"=3450, "滑动开关"=21011, "缓存级别数量"=24133, "换行符常量"=23501, "回车键常量"=23500, "回调事件引用句柄"=3435, "会话句柄至引用句柄转换"=2307, "混合复选框（系统）"=21333, "混合信号图"=21721, "获取帮助窗口状态"=1354, "获取变体属性"=8205, "获取波形成分"=2067, "获取波形属性"=8208, "获取菜单项信息"=9005, "获取定点分量"=11163, "获取队列引用"=9108, "获取队列状态"=9110, "获取记录数量"=8064, "获取矩阵对角"=8501, "获取矩阵元素"=8502, "获取卷信息"=8067, "获取快捷菜单信息"=9007, "获取权限"=8065, "获取日期/时间（秒）"=1303, "获取日期/时间字符串"=1600, "获取数据记录位置"=8061, "获取所选菜单项"=9001, "获取通知器引用"=9101, "获取通知器状态"=9103, "获取拖放数据"=9154, "获取文件大小"=8063, "获取文件类型和创建者"=8066, "获取文件位置"=8062, "获取子矩阵"=8503, "或"=1062, "或非"=1072, "基本单位转换"=1079, "极坐标至复数转换"=1047, "极坐标至实部虚部转换"=23061, "计算机Epsilon"=23528, "加"=1050, "加1"=1057, "加（带错误接线端）"=3915, "假常量"=2006, "检查结构类型是否匹配"=2416, "检查值"=3833, "简易垂直滑动杆"=3002, "简易数值"=2900, "简易水平滑动杆"=3003, "简易字符串"=2115, "减"=1051, "减1"=1058, "减（带错误接线端）"=3916, "交叉"=2197, "交换器"=3828, "交换向量元素"=1912, "交换值"=2401, "交换字"=1163, "交换字节"=1162, "交织一维数组"=2045, "接收数据"=1974, "截取字符串"=1503, "解除捆绑"=2048, "经典垂直滑动杆"=3004, "经典水平滑动开关"=3114, "经典颜色盒"=3013, "经典颜色梯度"=3022, "静态VI引用"=2084, "竞争结构"=2371, "旧VISA打开"=1921, "局部变量"=2061, "矩形停止按钮"=3128, "矩阵大小"=8507, "矩阵转置"=8509, "拒绝访问"=8057, "句柄存数"=1605, "句柄取数"=1604, "卷信息"=1414, "绝对值"=1054, "开关按钮"=21001, "可打印？"=1124, "空白？"=1125, "空路径常量"=23523, "空数组？"=23063, "空字符串/路径？"=1112, "空字符串常量"=23503, "控件引用句柄"=3419, "控件与仿真循环"=2099, "控制帮助窗口"=1353, "控制在线帮助"=1355, "捆绑"=2049, "蓝牙网络连接引用句柄"=3468, "类说明符常量"=2094, "类型"=2414, "类型必须为簇"=2418, "类型必须为数组"=2417, "类型错误"=2415, "类型和创建者"=1434, "类型专用结构"=2373, "里德伯常数(1/m)"=23521, "连接"=2195, "连接字符串"=2040, "量表（经典）"=3040, "量表（新式）"=21009, "列表框（经典）"=21806, "列表框（系统）"=21805, "列表框（新式）"=21792, "列表框符号下拉列表控件常量"=2038, "列表目录"=1418, "临时目录"=1435, "漏斗#1"=21754, "漏斗#2"=3072, "路径常量"=2009, "路径类型"=1421, "路径至字符串数组转换"=1423, "路径至字符串转换"=1077, "罗列文件夹"=8083, "逻辑移位"=1081, "枚举（经典）"=3023, "枚举（系统）"=3062, "枚举（新式）"=21605, "枚举常量"=2090, "秒至日期/时间转换"=1309, "摩尔气体常数(J/(mol K))"=23522, "默认目录"=1427, "内嵌C节点"=2104, "判定范围并强制转换"=1127, "匹配模式"=1535, "匹配真/假字符串"=1533, "匹配字符串"=1532, "平方"=23059, "平方根"=1060, "平滑的椭圆"=32500, "平滑的圆角矩形"=32505, "平化至JSON"=24201, "平化至XML"=8400, "平化至字符串"=1164, "平化字符串至变体转换"=8202, "平面反向三角形"=3623, "平面方形按钮"=3103, "平面盒"=3602, "平面框"=3608, "平面右向三角形"=3621, "平面圆盒"=3611, "平面圆形"=3605, "平面圆形按钮"=3102, "平面正向三角形"=3622, "平面左向三角形"=3620, "平铺式顺序结构"=2069, "平台平面方形按钮"=3134, "普朗克常数(J/Hz)"=23516, "启用本地模式"=1963, "启用菜单跟踪"=9002, "启用远程模式"=1964, "强度图（经典）"=3510, "强度图（新式）"=21720, "强度图表（经典）"=3509, "强度图表（新式）"=21719, "强制类型转换"=1166, "强制转换至类型"=2402, "翘板开关"=21002, "清除定点溢出状态"=5562, "清空队列"=9114, "清空事件队列"=2135, "请求释放内存"=1610, "区域"=2196, "取负数"=1069, "取消按钮（系统）"=3131, "取消按钮（新式）"=21739, "取消并行轮询配置"=1971, "取消释放变体值引用"=2411, "取消通知"=9107, "取消注册会话句柄"=2320, "取消注册事件"=2076, "全局变量"=2060, "确定按钮（系统）"=3130, "确定按钮（新式）"=21738, "日期/时间至秒转换"=1308, "三维图片"=23776, "扫描变量读取"=23784, "扫描变量写入"=23787, "扫描文件"=2082, "扫描值"=1534, "扫描字符串"=2080, "删除"=8056, "删除（过时）"=1417, "删除变体属性"=8206, "删除波形属性"=8209, "删除菜单项"=9004, "删除定点溢出状态"=5563, "删除数据值引用"=2409, "删除数组元素"=3912, "商与余数"=1056, "上矩形值（轮廓）"=21762, "上矩形值（平面）"=3702, "上矩形值（阴影）"=3802, "上凸反向三角形"=3615, "上凸盒（经典）"=3600, "上凸盒（新式）"=3637, "上凸框"=3606, "上凸右向三角形"=3613, "上凸圆盒"=3609, "上凸圆形"=3603, "上凸正向三角形"=3614, "上凸左向三角形"=3612, "设备控制/状态"=1433, "设备清零"=1961, "设备清零列表"=1962, "设备引用句柄"=3405, "设置RWLS"=1984, "设置变体属性"=8204, "设置波形属性"=8207, "设置菜单项信息"=9006, "设置超时"=1985, "设置记录数量"=8075, "设置矩阵对角"=8504, "设置矩阵元素"=8505, "设置句柄大小"=1603, "设置权限"=8076, "设置事件发生"=1702, "设置数据记录位置"=8072, "设置文件大小"=8074, "设置文件类型和创建者"=8077, "设置文件位置"=8073, "设置子矩阵"=8506, "生成地址"=1967, "十进制数？"=1119, "十进制数字符串至数值转换"=1184, "十六进制数？"=1123, "十六进制数字符串至数值转换"=1185, "时间标识（程序框图常量）"=2068, "时间标识输入控件（经典）"=5555, "时间标识输入控件（系统）"=21967, "时间标识输入控件（新式）"=21913, "时间标识显示控件（经典）"=5556, "时间标识显示控件（新式）"=21914, "时间计数器"=1300, "实部虚部至复数转换"=1046, "实部虚部至极坐标转换"=23060, "事件发生引用句柄"=3406, "事件回调注册"=2078, "事件结构"=2052, "事件数据节点"=2102, "释放变体值引用"=2410, "释放队列引用"=9109, "释放通知器引用"=9102, "首次调用？"=1083, "属性节点"=1920, "树形控件（经典）"=21819, "树形控件（系统）"=21794, "树形控件（新式）"=21793, "数据缓冲区大小"=24132, "数据记录文件引用句柄"=3402, "数据值引用"=3476, "数据值引用常量"=24134, "数值常量"=2005, "数值控件（经典）"=3000, "数值控件（系统）"=21919, "数值控件（新式）"=21003, "数值显示控件（经典）"=3001, "数值显示控件（新式）"=21004, "数值至八进制字符串转换"=1182, "数值至布尔数组转换"=1814, "数值至工程字符串转换"=1183, "数值至十进制数字符串转换"=1180, "数值至十六进制字符串转换"=1181, "数值至小数字符串转换"=1506, "数值至指数字符串转换"=1505, "数字波形图（经典）"=3511, "数字波形图（新式）"=21718, "数字数据（经典）"=3210, "数字数据（新式）"=21216, "数组（程序框图常量）"=2070, "数组（经典）"=3300, "数组（新式）"=21608, "数组插入"=3911, "数组大小"=1809, "数组内存信息"=2412, "数组元素或操作"=1910, "数组元素相乘"=1904, "数组元素相加"=1903, "数组元素与操作"=1911, "数组至比特包"=3136, "数组至簇转换"=1168, "数组至电子表格字符串转换"=1540, "数组子集"=2044, "数组最大值与最小值"=1907, "刷新流"=23808, "刷新文件"=8059, "刷新文件（过时）"=1406, "双按钮对话框"=1341, "双曲余割"=23053, "双曲余切"=23055, "双曲余弦"=1215, "双曲正割"=23054, "双曲正切"=1216, "双曲正弦"=1214, "水平按钮框"=3636, "水平分隔栏"=21861, "水平分隔栏（经典）"=21863, "水平分隔栏（系统）"=21865, "水平管道（平面）"=3810, "水平管道（阴影）"=3710, "水平罐"=3071, "水平滚动条"=21110, "水平滑动杆（经典）"=3010, "水平滑动杆（系统）"=21904, "水平进度条（系统）"=21910, "水平进度条（新式）"=21102, "水平开关"=3108, "水平刻度条"=21106, "水平平滑盒"=3633, "水平梯度矩形"=32504, "水平梯度椭圆"=32502, "水平梯度圆角矩形"=32507, "水平填充滑动杆（经典）"=3012, "水平填充滑动杆（新式）"=21100, "水平线"=3821, "水平摇杆开关（经典）"=3110, "水平摇杆开关（新式）"=21700, "水平指针滑动杆（经典）"=3011, "水平指针滑动杆（系统）"=21902, "水平指针滑动杆（新式）"=21101, "搜索"=1409, "搜索/拆分字符串"=1538, "搜索变量容器"=23802, "搜索红外线"=9141, "搜索蓝牙设备"=9152, "搜索替换字符串"=3914, "搜索一维数组"=1901, "随机数(0-1)"=1070, "索引数组"=2042, "索引与捆绑簇数组"=2056, "索引字符串数组"=1531, "锁定范围"=1411, "替换数组子集"=3910, "替换子字符串"=3913, "添加真/假字符串"=1511, "条件结构"=2001, "条件禁用结构"=2064, "停止"=1350, "停止按钮"=21230, "通过引用调用"=3901, "通过引用调用MathScript"=3906, "通知器引用句柄"=3423, "同或"=1073, "图片下拉列表（经典）"=3015, "图片下拉列表（系统）"=21925, "图片下拉列表（新式）"=21602, "退出LabVIEW"=1352, "尾数与指数"=1150, "未组合的矩阵"=23000, "温度计（经典）"=3021, "温度计（新式）"=21007, "文本按钮"=21015, "文本下拉列表（程序框图常量）"=2008, "文本下拉列表（经典）"=3014, "文本下拉列表（系统）"=3060, "文本下拉列表（新式）"=21601, "文本与图片下拉列表（经典）"=3016, "文本与图片下拉列表（新式）"=21603, "文本至UTF-8转换"=23066, "文件/目录信息"=8082, "文件/目录信息（过时）"=1413, "文件对话框"=8058, "文件对话框（过时）"=8081, "文件路径输入控件（经典）"=3203, "文件路径输入控件（系统）"=21922, "文件路径输入控件（新式）"=21730, "文件路径显示控件（经典）"=3204, "文件路径显示控件（新式）"=21731, "系统测试"=1987, "系统复位"=1976, "下凹菜单下拉列表"=3019, "下凹反向三角形"=3619, "下凹盒"=3601, "下凹盒（粗）"=3635, "下凹框（系统）"=3624, "下凹框（新式）"=3607, "下凹右向三角形"=3617, "下凹圆盒"=3638, "下凹圆盒 1"=3610, "下凹圆形"=3604, "下凹正向三角形"=3618, "下凹左向三角形"=3616, "下矩形值（轮廓）"=3806, "下矩形值（平面）"=3706, "下矩形值（阴影）"=21766, "下拉菜单下拉列表"=3061, "线条（粗）"=3629, "线条（分隔，粗）"=3630, "线条（分隔，系统）"=3632, "线条（分隔，细）"=3627, "线条（细）"=3626, "像素图"=3505, "像素图（警告：危险）"=3507, "向流中写入单个元素"=23798, "向流中写入多个元素"=23804, "向上T形（平面）"=3812, "向上T形（阴影）"=3712, "向上箭头"=3823, "向上箭头值（轮廓）"=3803, "向上箭头值（平面）"=3703, "向上箭头值（阴影）"=21763, "向上取整"=1076, "向下T形（平面）"=3818, "向下T形（阴影）"=3718, "向下箭头"=3824, "向下箭头值（轮廓）"=3807, "向下箭头值（平面）"=3707, "向下箭头值（阴影）"=21767, "向下取整"=1075, "向右T形（平面）"=3815, "向右T形（阴影）"=3715, "向右箭头值（轮廓）"=3805, "向右箭头值（平面）"=3705, "向右箭头值（阴影）"=21765, "向左T形（平面）"=3809, "向左T形（阴影）"=3709, "向左箭头值（轮廓）"=3801, "向左箭头值（平面）"=3701, "向左箭头值（阴影）"=21761, "销毁流端点"=23794, "销毁用户事件"=2075, "小于0？"=1118, "小于？"=1111, "小于等于0？"=1115, "小于等于？"=1104, "写入DataSocket"=1087, "写入TCP数据"=1714, "写入UDP数据"=1725, "写入变量"=23782, "写入变量（超时方式）"=23789, "写入二进制文件"=8078, "写入红外线数据"=9146, "写入蓝牙数据"=9150, "写入设备"=1431, "写入数据记录文件"=8079, "写入文本文件"=8080, "写入文件"=1408, "新建VI"=8014, "新建VI对象"=8015, "新建目录"=1402, "新建数据值引用"=2408, "新文件"=1404, "行结束常量"=23525, "修剪的边角矩形"=32513, "旋钮（经典）"=3005, "旋钮（新式）"=21000, "旋转供给器"=3830, "选项卡控件（NXG风格）"=32700, "选项卡控件（经典）"=3330, "选项卡控件（系统）"=3331, "选项卡控件（新式）"=3332, "选行并添加至字符串"=1510, "选择"=1516, "循环移位"=1082, "压力罐（平面）"=3075, "压力罐（阴影）"=21753, "压缩器"=3832, "颜色盒常量"=2120, "颜色盒窄边"=2905, "液罐（经典）"=3020, "液罐（新式）"=21006, "一维数组插值"=1905, "一维数组排序"=1120, "一维数组循环移位"=1906, "一维数组转置"=23068, "移动"=8068, "移动（过时）"=1415, "仪表（经典）"=3030, "仪表（新式）"=21008, "以10为底的e的对数"=23512, "以阈值插值一维数组"=1909, "异或"=1063, "引用句柄至会话句柄转换"=2306, "引用句柄至路径转换"=1424, "应用程序引用句柄"=3412, "用户定义标识符（程序框图常量）"=2114, "用户定义标识符（经典）"=3329, "用户定义标识符（新式）"=21749, "用户定义引用句柄"=3428, "用户定义引用句柄标识符（程序框图常量）"=3426, "用户定义引用句柄标识符（经典）"=3429, "用户定义引用句柄标识符（新式）"=21745, "用户定义引用句柄标识符平化（经典）"=3454, "用户定义引用句柄标识符平化（新式）"=21747, "用户项"=3506, "有损耗元素入队列"=9130, "右泵（平面）"=3819, "右泵（阴影）"=3719, "右箭头"=3825, "右矩形值（轮廓）"=3804, "右矩形值（平面）"=3704, "右矩形值（阴影）"=21764, "右上弯管（平面）"=3814, "右上弯管（阴影）"=3714, "右下弯管（平面）"=3817, "右下弯管（阴影）"=3717, "余割"=1204, "余切"=1205, "余弦"=1201, "与"=1061, "与非"=1071, "预分配的读取二进制文件"=24135, "预览队列元素"=9112, "元电荷(C)"=23517, "元素出队列"=9113, "元素入队列"=9111, "元素同址操作结构"=2360, "圆形按钮"=3100, "圆形单选按钮"=3106, "圆形灯"=3104, "圆形开关按钮"=3118, "圆形开关按钮（性能分析）"=3112, "圆形停止按钮"=3127, "圆形指示灯（经典）"=3120, "圆形指示灯（新式）"=21012, "运动资源（程序框图常量）"=3449, "运动资源（经典）"=3448, "运动资源（新式）"=21787, "蕴含"=1080, "在后台打开变量连接"=23791, "在字符串中搜索标记"=8101, "真空光速(m/sec)"=23518, "整数拼接"=1171, "整型转换为定点"=5567, "正割"=1203, "正切"=1202, "正无穷大"=23515, "正弦"=1200, "正弦与余弦"=1220, "直接变量读取"=23785, "直接变量写入"=23788, "指示灯按钮"=3116, "指数"=1211, "制表符常量"=23502, "终端结构"=2370, "重力常数(Nm2/kg2)"=23519, "重排数组维数"=2055, "重组变体（警告：危险）"=2405, "重组解锁数据变量引用（警告：危险）"=2407, "重组数组"=2403, "注册会话句柄"=2319, "注册事件"=2065, "转换为64位整型"=1155, "转换为OLE变体"=8002, "转换为变体"=8201, "转换为长整型"=1142, "转换为大写字母"=1188, "转换为单精度浮点数"=1146, "转换为单精度复数"=1151, "转换为单字节整型"=1140, "转换为定点数"=5561, "转换为扩展精度浮点数"=1149, "转换为扩展精度复数"=1154, "转换为时间标识"=5560, "转换为双精度浮点数"=1147, "转换为双精度复数"=1152, "转换为双字节整型"=1141, "转换为探针字符串"=2413, "转换为特定的类"=8016, "转换为通用的类"=8017, "转换为无符号64位整型"=1156, "转换为无符号长整型"=1145, "转换为无符号单字节整型"=1143, "转换为无符号双字节整型"=1144, "转换为小写字母"=1189, "转盘（经典）"=3050, "转盘（新式）"=21732, "状态"=2198, "状态图"=2051, "准备接收"=1975, "资源索引"=1088, "子面板"=21810, "子面板（经典）"=21811, "子面板（系统）"=21823, "自动化引用句柄"=3410, "自然对数"=1209, "自然对数 (Arg +1)"=1221, "自然对数的底数"=23510, "自由标签"=2321, "字符串常量"=2007, "字符串长度"=1502, "字符串输入控件（经典）"=3200, "字符串输入控件（系统）"=21920, "字符串输入控件（新式）"=21701, "字符串数组排序"=23065, "字符串数组至路径转换"=1422, "字符串显示控件（经典）"=3201, "字符串显示控件（新式）"=21702, "字符串移位"=1536, "字符串至IP地址转换"=1711, "字符串至共享变量转换"=1830, "字符串至路径转换"=1078, "字符串至字节数组转换"=1608, "字符类"=1126, "字节流文件引用句柄"=3408, "字节数组至字符串转换"=1609, "总是复制"=2400, "组合框（经典）"=3304, "组合框（系统）"=21917, "组合框（新式）"=21604, "组合框常量"=2088, "最大值与最小值"=1108, "最近数取整"=1055, "左泵（平面）"=3813, "左泵（阴影）"=3713, "左箭头"=3826, "左矩形值（轮廓）"=3800, "左矩形值（平面）"=3700, "左矩形值（阴影）"=21760, "左上弯管（平面）"=3808, "左上弯管（阴影）"=3708, "左下弯管（平面）"=3811, "左下弯管（阴影）"=3711]
            (unwired) "NumText.TextColor"
            n9 = property on="数值" class="DigNum (严格)"() -> ("Bounds"=w44:T4)  [unwired: 2 in, 2 out]
            n10 = New VI Object(vi object class=w49, owner refnum=w46, style=w51, position/next to=T3 {"Horizontal"=25, "Vertical"=250} ("位置"), 4:w44, 8:w48) -> (object refnum=w45:refnum<vi>)  [unwired: 2 in, 1 out]
          }
        }
        n11 = To More Specific Class(target class=w36, reference=w28, error in=w33) -> (specific class reference=w35:refnum<vi>, error out=w32:errorcluster)
        n12 = property class="DigNum"(reference=w35, error in=w32) -> ("NumText.TextColor"=w34:u32, "NumText.Size"=w21:T4, "NumText.Font"=w20:T5, "Text Width"=w19:u32)  [unwired: 2 out]
        n13 = local read item#-1() -> (w26)
        n14 = property class="DigNum"(reference=w23, "NumText.BGColor"=u32 16777216 ("数值文本.文本颜色:背景色"), "NumText.TextColor"=w26, "NumText.Size"=w21, "NumText.Font"=w20, "Text Width"=w19) -> (reference out=w24:refnum<vi>)  [unwired: 1 in, 1 out]
        n15 = Wait (ms)(milliseconds to wait=u32 200 ("等待时间（毫秒）")) -> ()  [unwired: 1 out]
      }
      n16 = invoke class="DigNum" method="Delete"(reference=w17) -> ()  [unwired: 2 in, 3 out]
    }
    frame Enabled {
    }
  }
  n17 = call <vilib>:"SA Set Panes Origin.vi"("Enable? (F)"=TRUE, "VI Ref in"=w13) -> ("VI Ref out"=w14:refnum<vi>)  [unwired: 9 in]
  n18 = call "MainDataStructure.vi"() -> ("Data Structure"=w1:T7)
  n19 = Bundle By Name(cluster=w1, "All Ref.VIRef"=w14, "Main VI.Main Name"=w9, "Error"=w6) -> (w7:T7)
  n20 = while {
    shift-right: [w52] -> w2
    shift-left: w7 -> [w57]
    shift-right: [w58] -> _
    shift-left: string[] ["MV :Core - Initialize", "MV :Core - Initialize System Path", "MV :Core - Initialize Thread Path", "MV :Core - Initialize Ref", "MV :Core - Initialize Data"] -> [w61]
    tunnel: "MV :Core - Error Handle" ("Error Handle") -> [w54]
    stop <- w55 stop-if-true
    # "SW Architecture - Consumer Loop - Respone Command and Build New Threads"
    n21 = Unbundle By Name(w57) -> ("Error"=w56:errorcluster)
    n22 = call <vilib>:"SA Get Next Event.vi"("Error Handle"=w54, "error in"=w56, "event queue in"=w61) -> ("prev event"=w53:string, "next event"=w60:string, "event queue out"=w59:string[])  [unwired: 6 in]
    "Current State" <- w60
    n23 = case shown="\"MV :Actn - CreateCotrl\"" w60 {
      tunnel: w57 -> [w62 w64 w87 w94 w113 w131 w140 w150 w159 w163 w171 w183 w197 w207 w221 w232 w244 w268 w279 w287 w292 w294 w299 w301 w306 w314 w323 w335 w357 w369 w391 w413 w428 w429 w434 w441 w486 w495 w504 w508 w527 w535 w543 w549]
      tunnel: w59 -> [w63 w74 w89 w95 w114 w132 w141 w151 w162 w164 w177 w190 w203 w214 w222 w233 w251 w277 w286 w288 w290 w295 w297 w302 w304 w312 w321 w333 w355 w367 w389 w411 w426 w430 w432 w447 w484 w493 w502 w519 w525 w533 w541 w547]
      tunnel: [w63 w73 w89 w91 w114 w132 w141 w151 w157 w164 w177 w190 w203 w204 w219 w233 w251 w277 w286 w288 w289 w295 w296 w302 w303 w311 w320 w332 w354 w366 w388 w410 w425 w430 w431 w446 w483 w492 w501 w518 w524 w532 w540 w546] -> w58
      tunnel: [w62 w75 w88 w93 w112 w130 w138 w149 w160 w163 w169 w181 w195 w206 w220 w231 w243 w267 w278 w287 w291 w294 w298 w301 w305 w313 w322 w334 w356 w368 w390 w412 w427 w429 w433 w448 w485 w494 w503 w507 w526 w534 w542 w548] -> w52
      tunnel: w53 -> [_ _ w77 _ _ _ _ _ _ _ _ _ _ _ _ _ _ _ _ _ _ _ _ _ _ _ _ _ _ _ _ _ _ _ _ _ _ _ _ _ _ _ _ _]
      frame "----------Core Status----------" {
      }
      frame "MV :Core - No Action", Default {
        n24 = Unbundle By Name(w64) -> ("Main VI.Main Name"=w67:string, "Error"=w71:errorcluster)
        n25 = Unbundle By Name(w64) -> ("Dynamic Threads Array"=→"Dynamic Threads Array":string[])
        n26 = call <vilib>:"SA Remove Queue Element.vi"("Time out (10)"=20 ("Time out(-1)_queue out"), "error in"=w71, "Queue Name"=w67) -> ("error out"=w70:errorcluster, "Data"=w69:variant, "Event"=w68:string)  [unwired: 5 in, 1 out]
        n27 = Build Array (concatenate)(w74, w68) -> (w73:string[])
        n28 = Bundle By Name(cluster=w64, "Main VI.Main Data"=w69, "Error"=w70) -> (w75:T7)
        n29 = Wait (ms)(milliseconds to wait=u32 50 ("等待时间（毫秒）")) -> ()  [unwired: 1 out]
      }
      frame "MV :Core - Error Handle" {
        w76 = T10 0 items=["no dialog", "OK message", "continue or stop message", "OK message + warnings", "continue/stop + warnings"] ("type of dialog (OK msg:1)")
        w84 = T10 2 items=["no dialog", "OK message", "continue or stop message", "OK message + warnings", "continue/stop + warnings"] ("type of dialog (OK msg:1)")
        n30 = Unbundle By Name(w87) -> ("Error.source"=w78:string, "Error"=w81:errorcluster)
        n31 = call <vilib>:"Simple Error Handler.vi"("type of dialog (OK msg:1)"=w76, "error in (no error)"=w81) -> ("error out"=w80:errorcluster, "message"=w79:string)  [unwired: 3 in, 3 out]
        n32 = Concatenate Strings(w77, " -> " ("字符串"), w78, w79) -> (→"Error Report":string)
        n33 = call <vilib>:"Simple Error Handler.vi"("type of dialog (OK msg:1)"=w84, "error in (no error)"=w80) -> ("error out"=w86:errorcluster)  [unwired: 3 in, 4 out]
        n34 = call <vilib>:"Clear Errors.vi"("error in (no error)"=w86) -> ("error out"=w85:errorcluster)  [unwired: 5 in, 1 out]
        n35 = Bundle By Name(cluster=w87, "Error"=w85) -> (w88:T7)
      }
      frame "MV :Core - Initialize" {
        n36 = Unbundle By Name(w94) -> ("Main VI.Main Name"=w92:string)  [unwired: 1 out]
        n37 = Bundle By Name(cluster=w94, "Thread to Operate.Queue Info.HighLevel Thread"=w92) -> (w93:T7)
        n38 = Build Array (concatenate)(w95, string[] [] ("数组")) -> (w91:string[])
      }
      frame "MV :Core - Initialize System Path" {
        w99 = "InNameLable.xls" ("Run Time relative path")
        w98 = 1 ("Development File Depth")
        w103 = "Reentrant VI Invoked by MainVI.vi" ("Run Time relative path")
        w102 = 1 ("Development File Depth")
        w107 = "Engine.vi" ("Run Time relative path")
        w106 = 1 ("Development File Depth")
        w108 = "Thread Invoked by MainVI.vi" ("Run Time relative path")
        w110 = 1 ("Development File Depth")
        n39 = Current VI's Path() -> (path=w97:path)
        n40 = Current VI's Path() -> (path=w111:path)
        n41 = Current VI's Path() -> (path=w101:path)
        n42 = Current VI's Path() -> (path=w105:path)
        n43 = call <vilib>:"SA Relative Path.vi"("Development Relative Path"=w99, "Run Time Relative path"=w99, "Run-Time File Depth"=w98, "Development File Depth"=w98, "Root Path"=w97) -> ("Relative Path"=w96:path)  [unwired: 5 in, 1 out]
        n44 = call <vilib>:"SA Relative Path.vi"("Development Relative Path"=w108, "Run Time Relative path"=w108, "Run-Time File Depth"=w110, "Development File Depth"=w110, "Root Path"=w111) -> ("Relative Path"=w109:path)  [unwired: 5 in, 1 out]
        n45 = call <vilib>:"SA Relative Path.vi"("Development Relative Path"=w103, "Run Time Relative path"=w103, "Run-Time File Depth"=w102, "Development File Depth"=w102, "Root Path"=w101) -> ("Relative Path"=w100:path)  [unwired: 5 in, 1 out]
        n46 = call <vilib>:"SA Relative Path.vi"("Development Relative Path"=w107, "Run Time Relative path"=w107, "Run-Time File Depth"=w106, "Development File Depth"=w106, "Root Path"=w105) -> ("Relative Path"=w104:path)  [unwired: 5 in, 1 out]
        n47 = Bundle By Name(cluster=w113, "界面控件.名称列表路径"=w96, "Dynamic VI Path.Thread Path"=w109, "Reentrant VI Path.Reentrant Thread Path"=w100, "Engine Path.Engine Path"=w104) -> (w112:T7)
      }
      frame "MV :Core - Initialize Thread Path" {
        w122 = "Reentrant VI Invoked by MainVI.vi" ("Run Time relative path")
        w121 = 1 ("Development File Depth")
        w126 = "Engine.vi" ("Run Time relative path")
        w125 = 1 ("Development File Depth")
        w127 = "Thread Invoked by MainVI.vi" ("Run Time relative path")
        w129 = 1 ("Development File Depth")
        n48 = Current VI's Path() -> (path=w118:path)
        n49 = for {
          tunnel: w118 -> [w136]
          tunnel: string[] ["..\\DynamicThreads\\ReOrigin.vi"] -> [w135] mode=indexing
          tunnel: [w133] -> w116 mode=indexing
          w134 = 1 ("Development File Depth")
          n50 = call <vilib>:"SA Relative Path.vi"("Development Relative Path"=w135, "Run Time Relative path"=w135, "Run-Time File Depth"=w134, "Development File Depth"=w134, "Root Path"=w136) -> ("Relative Path"=w133:path)  [unwired: 5 in, 1 out]
        }
        n51 = Current VI's Path() -> (path=w120:path)
        n52 = Current VI's Path() -> (path=w124:path)
        n53 = Index Array(array=w116) -> (element=w115:path)  [unwired: 1 in]
        n54 = call <vilib>:"SA Relative Path.vi"("Development Relative Path"=w127, "Run Time Relative path"=w127, "Run-Time File Depth"=w129, "Development File Depth"=w129, "Root Path"=w118) -> ("Relative Path"=w128:path)  [unwired: 5 in, 1 out]
        n55 = call <vilib>:"SA Relative Path.vi"("Development Relative Path"=w122, "Run Time Relative path"=w122, "Run-Time File Depth"=w121, "Development File Depth"=w121, "Root Path"=w120) -> ("Relative Path"=w119:path)  [unwired: 5 in, 1 out]
        n56 = call <vilib>:"SA Relative Path.vi"("Development Relative Path"=w126, "Run Time Relative path"=w126, "Run-Time File Depth"=w125, "Development File Depth"=w125, "Root Path"=w124) -> ("Relative Path"=w123:path)  [unwired: 5 in, 1 out]
        n57 = Bundle By Name(cluster=w131, "DynamicThreadsPath.ReOriginVI"=w115, "Dynamic VI Path.Thread Path"=w128, "Reentrant VI Path.Reentrant Thread Path"=w119, "Engine Path.Engine Path"=w123) -> (w130:T7)
      }
      frame "MV :Core - Initialize Ref" {
        n58 = Unbundle By Name(w140) -> ("Error"=w139:errorcluster)
        n59 = control-ref of="界面控件"() -> (w137:refnum<vi>)
        n60 = Bundle By Name(cluster=w140, "All Ref.界面控件Ref"=w137, "Error"=w139) -> (w138:T7)
      }
      frame "MV :Core - Initialize Data" {
        n61 = Unbundle By Name(w150) -> ("All Ref.界面控件Ref"=w148:refnum<vi>, "Error"=w146:errorcluster)
        n62 = property class="Clust (严格)"(reference=w148, error in=w146) -> (error out=w145:errorcluster, "Value"=w147:T2)  [unwired: 1 out]
        n63 = Unbundle By Name(w147) -> ("颜色盒"=w144:u32, "VI路径"=w143:path, "控件名称"=w142:string)
        n64 = Bundle By Name(cluster=w150, "Error"=w145, "界面控件.颜色盒"=w144, "界面控件.当前选择路径"=w143, "界面控件.控件名称"=w142) -> (w149:T7)
      }
      frame "MV :Core - Exit System" {
        n65 = Unbundle By Name(w159) -> ("Dynamic Threads Array"=w158:string[], "Error"=w161:errorcluster)
        n66 = Wait (ms)(milliseconds to wait=u32 10 ("等待时间（毫秒）")) -> ()  [unwired: 1 out]
        n67 = local write "Dynamic Threads Array"(w158) -> ()
        n68 = Empty Array?(array=w158) -> (empty?=w153:bool)
        n69 = Select(t=string[] [], s=w153, f=string[] ["MV :Core - Exit System"]) -> (s? t:f=w155:string[])
        n70 = Build Array (concatenate)(w162, w155) -> (w157:string[])
        n71 = Bundle By Name(cluster=w159, "Exit"=w153, "Error"=w161) -> (w160:T7)
      }
      frame "----------Thread Manage----------" {
      }
      frame "MV :TM - Load Dynamic VI" {
        n72 = Unbundle By Name(w171) -> ("Dynamic Threads Array"=w173:string[], "Thread to Operate.Queue Info.Thread Q Name"=w165:string, "Thread to Operate.Invoke Property"=w166:T9, "Thread to Operate.Thread VI Path"=w172:path, "Thread to Operate.Queue Info"=w167:T11, "Error"=w174:errorcluster)
        n73 = call <vilib>:"SA Dynamic Call_Single.vi"("Invoke Property"=w166, "error in (no error)"=w174, "Queue Info"=w167, "vi path"=w172) -> ("error out"=w170:errorcluster, "call failed"=w175:bool)  [unwired: 5 in, 1 out]
        n74 = Build Array (concatenate)(w173, w165) -> (w176:string[])
        n75 = Select(t=w173, s=w175, f=w176) -> (s? t:f=w168:string[])
        n76 = Bundle By Name(cluster=w171, "Dynamic Threads Array"=w168, "Error"=w170) -> (w169:T7)
      }
      frame "MV :TM - Load Engine" {
        n77 = Unbundle By Name(w183) -> ("Dynamic Threads Array"=w186:string[], "Thread to Operate.Queue Info.Thread Q Name"=w185:string, "Thread to Operate.Invoke Property"=w179:T9, "Thread to Operate.Thread VI Path"=w184:path, "Thread to Operate.Queue Info"=w178:T11, "Error"=w187:errorcluster)
        n78 = call <vilib>:"SA Dynamic Call_Single.vi"("Invoke Property"=w179, "error in (no error)"=w187, "Queue Info"=w178, "vi path"=w184) -> ("error out"=w182:errorcluster, "call failed"=w188:bool)  [unwired: 5 in, 1 out]
        n79 = Build Array (concatenate)(w186, w185) -> (w189:string[])
        n80 = Select(t=w186, s=w188, f=w189) -> (s? t:f=w180:string[])
        n81 = Bundle By Name(cluster=w183, "Dynamic Threads Array"=w180, "Error"=w182) -> (w181:T7)
      }
      frame "MV :TM - Load Reentrant VI" {
        n82 = Unbundle By Name(w197) -> ("Dynamic Threads Array"=w199:string[], "Thread to Operate.Queue Info.Thread Q Name"=w192:string, "Thread to Operate.Invoke Property"=w191:T9, "Thread to Operate.Thread VI Path"=w198:path, "Thread to Operate.Queue Info"=w193:T11, "Error"=w200:errorcluster)
        n83 = call <vilib>:"SA Dynamic Call_Single.vi"("Invoke Property"=w191, "error in (no error)"=w200, "Queue Info"=w193, "vi path"=w198) -> ("error out"=w196:errorcluster, "call failed"=w201:bool)  [unwired: 5 in, 1 out]
        n84 = Build Array (concatenate)(w199, w192) -> (w202:string[])
        n85 = Select(t=w199, s=w201, f=w202) -> (s? t:f=w194:string[])
        n86 = Bundle By Name(cluster=w197, "Dynamic Threads Array"=w194, "Error"=w196) -> (w195:T7)
      }
      frame "MV :TM - Clean Dynamic Thread" {
        n87 = Unbundle By Name(w207) -> ("Thread to Operate.Queue Info.Thread Q Name"=w208:string)
        n88 = To Variant(anything=TRUE) -> (Variant=w211:variant)
        n89 = Build Array(w208) -> (w213:string[])
        n90 = Build Array("TM :THx - Quit Dynamic Thread") -> (w209:string[])
        n91 = Build Array(w211) -> (w210:variant[])
        n92 = Bundle By Name(cluster=w207, "Send Data to Thread.Thread to Send"=w213, "Send Data to Thread.Order to Send"=w209, "Send Data to Thread.Data to Send"=w210) -> (w206:T7)
        n93 = Build Array (concatenate)(w214) -> (w204:string[])
      }
      frame "MV :TM - Clean All Dynamic Thread" {
        n94 = Unbundle By Name(w221) -> ("Dynamic Threads Array"=w218:string[])
        n95 = Array Size(array=w218) -> (size(s)=w216:i32)
        n96 = Initialize Array("TM :THx - Quit Dynamic Thread", w216) -> (w215:string[])
        n97 = Build Array (concatenate)(w222) -> (w219:string[])
        n98 = Bundle By Name(cluster=w221, "Send Data to Thread.Thread to Send"=w218, "Send Data to Thread.Order to Send"=w215) -> (w220:T7)
      }
      frame "MV :TM - Shut Down Threads" {
        n99 = Unbundle By Name(w232) -> ("Dynamic Threads Array"=w224:string[], "Send Data to Thread.Thread to Send"=w225:string[], "Send Data to Thread.Order to Send"=w226:string[], "Send Data to Thread.Data to Send"=w227:variant[], "Error"=w229:errorcluster)
        n100 = call <vilib>:"SA Dynamic Thread Close By Order.vi"("error in (no error)"=w229, "datas of quit"=w227, "commands of quit"=w226, "command queue names"=w225) -> ("error out"=w228:errorcluster, "close failed"=w230:bool[])  [unwired: 5 in, 1 out]
        n101 = for {
          tunnel: w230 -> [w234] mode=indexing
          tunnel: w225 -> [w237] mode=indexing
          shift-right: [w235] -> w223
          shift-left: w224 -> [w236]
          n102 = case shown="真" w234 {
            tunnel: w237 -> [_ w239]
            tunnel: w236 -> [w238 w242]
            tunnel: [w238 w241] -> w235
            frame False {
            }
            frame True {
              n103 = Search 1D Array(1D array=w242, element=w239) -> (index of element=w240:i32)  [unwired: 1 in]
              n104 = Delete From Array(array=w242, index=w240) -> (array with subset deleted=w241:string[])  [unwired: 1 in, 1 out]
            }
          }
        }
        n105 = Bundle By Name(cluster=w232, "Dynamic Threads Array"=w223, "Error"=w228) -> (w231:T7)
      }
      frame "MV :TM - Send To Threads" {
        n106 = Unbundle By Name(w244) -> ("Send Data to Thread.Thread to Send"=w250:string[], "Send Data to Thread.Order to Send"=w248:string[], "Send Data to Thread.Data to Send"=w247:variant[], "Error"=w249:errorcluster)
        n107 = for {
          tunnel: w250 -> [w257] mode=indexing
          tunnel: w249 -> [w260]
          tunnel: w248 -> [w259]
          tunnel: w247 -> [w258]
          tunnel: [w253] -> w246 mode=indexing
          i -> [w252]
          n108 = call <vilib>:"SA Verify Queue.vi"("Queue Name in"=w257) -> ("Not A Queue?"=w256:bool)  [unwired: 6 in, 3 out]
          n109 = Index Array(array=w259, index=w252) -> (element=w255:string)
          n110 = Index Array(array=w258, index=w252) -> (element=w254:variant)
          n111 = case shown="假" w256 {
            tunnel: w260 -> [w264 w266]
            tunnel: w257 -> [w261 _]
            tunnel: w255 -> [w263 _]
            tunnel: w254 -> [w262 _]
            tunnel: [w265 w266] -> w253
            frame False {
              n112 = call <vilib>:"SA Insert to Queue.vi"("error in"=w264, "Data"=w262, "Event"=w263, "Queue Name"=w261) -> ("error out"=w265:errorcluster)  [unwired: 7 in]
            }
            frame True {
            }
          }
        }
        n113 = Merge Errors(w246) -> (w245:errorcluster)
        n114 = Bundle By Name(cluster=w244, "Error"=w245) -> (w243:T7)
      }
      frame "THx :TM - Delete Dynamic Thread" {
        n115 = Unbundle By Name(w268) -> ("Dynamic Threads Array"=w273:string[], "Main VI.Main Order"=w274:string, "Main VI.Main Data"=w275:variant, "Error"=w276:errorcluster)
        n116 = Variant To Data(error in=w276, type=w274, Variant=w275) -> (data=w272:string, error out=w269:errorcluster)
        n117 = Search 1D Array(1D array=w273, element=w272) -> (index of element=w271:i32)  [unwired: 1 in]
        n118 = Delete From Array(array=w273, index=w271) -> (array with subset deleted=w270:string[])  [unwired: 1 in, 1 out]
        n119 = Bundle By Name(cluster=w268, "Dynamic Threads Array"=w270, "Error"=w269) -> (w267:T7)
      }
      frame "THx :TM - Return Error" {
        n120 = Unbundle By Name(w279) -> ("Error"=w283:errorcluster, "Main VI.Main Data"=w284:variant, "Error"=w285:errorcluster)
        n121 = Variant To Data(error in=w285, type=w283, Variant=w284) -> (data=w282:errorcluster, error out=w281:errorcluster)
        n122 = Merge Errors(w282, w281) -> (w280:errorcluster)
        n123 = Bundle By Name(cluster=w279, "Error"=w280) -> (w278:T7)
      }
      frame "----------Send (MV to THx)----------" {
      }
      frame "MV :THx - /* ADD NAME */" {
        n124 = Unbundle By Name(w292) -> ("Error"=w293:errorcluster)
        n125 = Build Array (concatenate)(w290) -> (w289:string[])
        n126 = Bundle By Name(cluster=w292, "Error"=w293) -> (w291:T7)
      }
      frame "----------Respond (THx to MV)----------" {
      }
      frame "THx :MV - /* ADD NAME */" {
        n127 = Unbundle By Name(w299) -> ("Error"=w300:errorcluster)
        n128 = Build Array (concatenate)(w297) -> (w296:string[])
        n129 = Bundle By Name(cluster=w299, "Error"=w300) -> (w298:T7)
      }
      frame "----------Action----------" {
      }
      frame "MV :Actn - /* ADD NAME */" {
        n130 = Unbundle By Name(w306) -> ("Error"=w307:errorcluster)
        n131 = Build Array (concatenate)(w304) -> (w303:string[])
        n132 = Bundle By Name(cluster=w306, "Error"=w307) -> (w305:T7)
      }
      frame "MV :Actn - OpenCtrlNameExcel" {
        n133 = Unbundle By Name(w314) -> ("界面控件.名称列表路径"=w309:path, "Error"=w310:errorcluster)
        n134 = call "OpenExcel.vi"("error in (no error)"=w310, "输入Excel路径"=w309) -> ("error out"=w308:errorcluster)  [unwired: 2 in]
        n135 = Build Array (concatenate)(w312) -> (w311:string[])
        n136 = Bundle By Name(cluster=w314, "Error"=w308) -> (w313:T7)
      }
      frame "MV :Actn - GetVICotrlName" {
        n137 = Unbundle By Name(w323) -> ("界面控件.当前选择路径"=w319:path, "Error"=w318:errorcluster)  [unwired: 1 out]
        n138 = call "获取VI中指定条件的控件名称列表.vi"("名称包含"=string[] ["TW0038", "TW0039"], "错误输入（无错误）"=w318, "路径"=w319) -> ("错误输出"=w317:errorcluster, "名称列表"=w316:string[])  [unwired: 6 in, 1 out]
        n139 = Bundle By Name(cluster=w323, "界面控件.名称列表"=w316, "Error"=w317) -> (w322:T7)
        n140 = Build Array (concatenate)(w321) -> (w320:string[])
      }
      frame "MV :Actn - WriteCtrlNameToExcel" {
        n141 = Unbundle By Name(w335) -> ("界面控件.名称列表路径"=w331:path, "界面控件.名称列表"=w330:string[], "Error"=w329:errorcluster)
        n142 = call-poly <vilib>:"Read Delimited Spreadsheet.vi"("file path (dialog if empty)"=w331) -> ("new file path (Not A Path if cancelled)"=w326:path, "all rows"=w324:string[][])  [unwired: 9 in, 4 out]
        n143 = Empty Array?(array=w324) -> (empty?=w325:bool)
        n144 = case shown="假" w325 {
          tunnel: w330 -> [w340 w342]
          tunnel: w329 -> [w339 w348]
          tunnel: [w338 w347] -> w328
          tunnel: w326 -> [w336 w345]
          tunnel: w324 -> [_ w344]
          frame True {
            n145 = call-poly <vilib>:"Write Delimited Spreadsheet.vi"("file path (dialog if empty)"=w336, "1D data"=w340, "error in (no error)"=w339, "transpose? (no:F)"=TRUE) -> ("error out"=w338:errorcluster)  [unwired: 10 in, 1 out]
          }
          frame False {
            n146 = Index Array(array=w344) -> (element=w343:string[])  [unwired: 2 in]
            n147 = Build Array(w343, w342) -> (w341:string[][])
            n148 = call-poly <vilib>:"Write Delimited Spreadsheet.vi"("file path (dialog if empty)"=w345, "2D data"=w341, "error in (no error)"=w348, "transpose? (no:F)"=TRUE) -> ("error out"=w347:errorcluster)  [unwired: 10 in, 1 out]
          }
        }
        n149 = Build Array (concatenate)(w333, string[] ["MV :Actn - OpenCtrlNameExcel"] ("数组")) -> (w332:string[])
        n150 = Bundle By Name(cluster=w335, "Error"=w328) -> (w334:T7)
      }
      frame "MV :Actn - ReOrigin" {
        n151 = Unbundle By Name(w357) -> ("Main VI.Main Data"=w351:variant, "Error"=w353:errorcluster)
        n152 = Variant To Data(error in=w353, type=T3 {"Horizontal"=0, "Vertical"=0} ("控件排布前面板.位置_前.位置"), Variant=w351) -> (data=w350:T3, error out=w352:errorcluster)
        n153 = Build Array (concatenate)(w355) -> (w354:string[])
        n154 = Bundle By Name(cluster=w357, "控件排布前面板.位置_前.位置"=w350, "Error"=w352) -> (w356:T7)
      }
      frame "MV :Actn - GetCotrlNameLable" {
        n155 = Current VI's Path() -> (path=w365:path)
        n156 = Strip Path(path=w365) -> (stripped path=w364:path)  [unwired: 1 out]
        n157 = Unbundle By Name(w369) -> ("Error"=w360:errorcluster)
        n158 = Build Path(base path=w364, name or relative path="lNameLable.xls" ("名称或相对路径")) -> (appended path=w361:path)
        n159 = Not A Number/Path/Refnum?(number/path/refnum=w361) -> (NaN/Path/Refnum?=w362:bool)
        n160 = case shown="假" w362 {
          tunnel: w361 -> [w375 _]
          tunnel: w360 -> [w374 w377]
          tunnel: [w371 w377] -> w359
          tunnel: [w370 string[] [] ("all rows")] -> w358
          frame False {
            n161 = call-poly <vilib>:"Read Delimited Spreadsheet.vi"("file path (dialog if empty)"=w375, "error in (no error)"=w374) -> ("all rows"=w373:string[][], "error out"=w371:errorcluster)  [unwired: 8 in, 4 out]
            n162 = Index Array(array=w373, index (col)=0 ("禁用的索引 (列)")) -> (element=w370:string[])  [unwired: 1 in]
          }
          frame True {
            n163 = One Button Dialog(message="未找到lNameLable.xls" ("消息")) -> ()  [unwired: 1 in, 1 out]
          }
        }
        n164 = Bundle By Name(cluster=w369, "控件排布前面板.lNameLable"=w358, "Error"=w359) -> (w368:T7)
        n165 = Build Array (concatenate)(w367) -> (w366:string[])
      }
      frame "MV :Actn - CreateCotrl" {
        n166 = Unbundle By Name(w391) -> ("控件排布前面板.获取引用.获取Ctl引用句柄"=w386:refnum<vi>, "控件排布前面板.获取引用.获取VI引用句柄"=w387:refnum<vi>, "控件排布前面板.lNameLable"=w384:string[], "Error"=w385:errorcluster, "控件排布前面板.位置_前.位置"=w382:T3)
        n167 = call "CreateCotrl.vi"("创建数量"="创建数量", "Position"=w382, "重置原点"=TRUE, "错误输入（无错误）"=w385, "lNameLable"=w384, "获取VI引用句柄"=w387, "Control输入"=w386) -> ("错误输出"=w381:errorcluster)
        n168 = flat-sequence {
          tunnel: w381 -> [w396]
          tunnel: [w396] -> w380
          tunnel: "创建数量" -> [w394]
          frame #0 {
            n169 = Number To Decimal String(number=w394) -> (decimal integer string=w393:string)  [unwired: 1 in]
            n170 = Concatenate Strings(w393, "个控件已创建完成！" ("字符串")) -> (w395:string)
            n171 = call "报警弹出信息.vi"("Diaplay Info"=w395) -> ()  [unwired: 10 in, 1 out]
          }
        }
        n172 = Build Array (concatenate)(w389) -> (w388:string[])
        n173 = Bundle By Name(cluster=w391, "Error"=w380) -> (w390:T7)
      }
      frame "MV :Actn - GetCotrlRef" {
        n174 = Unbundle By Name(w413) -> ("界面控件.当前选择路径"=w399:path, "Error"=w401:errorcluster, "界面控件.控件名称"=w398:string)  [unwired: 1 out]
        n175 = Open VI Reference(vi path=w399, error in (no error)=w401) -> (vi reference=w407:refnum<vi>, error out=w408:errorcluster)  [unwired: 4 in]
        n176 = property class="VI"(reference=w407, error in=w408, "Edit Mode"=TRUE ("以编辑模式打开")) -> (reference out=w403:refnum<vi>, error out=w409:errorcluster, "Panel"=w406:refnum<vi>)
        n177 = property class="Pnl"(reference=w406, error in=w409) -> (error out=w404:errorcluster, "Controls[]"=w405:refnum<vi>[])  [unwired: 1 out]
        n178 = for {
          tunnel: w405 -> [w419] mode=indexing
          tunnel: [w417] -> w402 if=w416
          shift-right: [w415] -> w400
          shift-left: w404 -> [w420]
          tunnel: w398 -> [w414]
          n179 = property class="Ctl"(reference=w419, error in=w420) -> (reference out=w417:refnum<vi>, error out=w415:errorcluster, "Label.Text"=w418:string)
          n180 = Equal?(x=w418, y=w414) -> (x = y?=w416:bool)
        }
        n181 = Bundle By Name(cluster=w413, "控件排布前面板.获取引用.获取VI引用句柄"=w403, "控件排布前面板.获取引用.获取Ctl引用句柄"=w402, "Error"=w400) -> (w412:T7)
        n182 = Build Array (concatenate)(w411) -> (w410:string[])
      }
      frame "MV :Actn - Open Front Panel" {
        n183 = Unbundle By Name(w428) -> ("All Ref.VIRef"=w424:refnum<vi>, "Error"=w423:errorcluster)
        n184 = invoke class="VI" method="FP.Open"(reference=w424, error in=w423, "State"=T8."Standard" ("状态")) -> (error out=w422:errorcluster)  [unwired: 2 in, 4 out]
        n185 = Build Array (concatenate)(w426) -> (w425:string[])
        n186 = Bundle By Name(cluster=w428, "Error"=w422) -> (w427:T7)
      }
      frame "----------Respond UI Events----------" {
      }
      frame "UI :Resp - /* ADD NAME */" {
        n187 = Unbundle By Name(w434) -> ("Error"=w435:errorcluster)
        n188 = Build Array (concatenate)(w432) -> (w431:string[])
        n189 = Bundle By Name(cluster=w434, "Error"=w435) -> (w433:T7)
      }
      frame "UI :Resp - PlanCtrlChange" {
        # "对界面上控件更新时，进行相应更新操作"
        n190 = Unbundle By Name(w441) -> ("Main VI.Main Data"=w444:variant, "Error"=w445:errorcluster)
        n191 = Variant To Data(error in=w445, type=cluster{refnum<vi>, "index of element":i32} {refnum, "index of element"=0} ("输出簇"), Variant=w444) -> (data=w443:cluster{refnum<vi>, "index of element":i32}, error out=w442:errorcluster)
        n192 = Unbundle(w443) -> (w436:refnum<vi>, "index of element"=w437:i32)
        n193 = case shown="2" w437 {
          tunnel: w442 -> [w457 w460 w472 w481]
          tunnel: w436 -> [w449 _ w464 w473]
          tunnel: [w453 w458 w468 w477] -> w440
          tunnel: w441 -> [w456 w463 w471 w480]
          tunnel: [w455 w462 w470 w479] -> w439
          frame 0, Default {
            n194 = property class="Ctl"(reference=w449, error in=w457) -> (error out=w454:errorcluster, "Value"=w452:variant)  [unwired: 1 out]
            n195 = Variant To Data(error in=w454, type=u32 0, Variant=w452) -> (data=w450:u32, error out=w453:errorcluster)
            n196 = Bundle By Name(cluster=w456, "界面控件.颜色盒"=w450) -> (w455:T7)
          }
          frame 1 {
            n197 = control-ref of="下拉列表"() -> (w461:refnum<vi>)
            n198 = property class="Ring (严格)"(reference=w461, error in=w460) -> (error out=w458:errorcluster, "RingText.Text"=w459:string)  [unwired: 1 out]
            n199 = Bundle By Name(cluster=w463, "界面控件.类名"=w459) -> (w462:T7)
          }
          frame 2 {
            n200 = property class="Ctl"(reference=w464, error in=w472) -> (error out=w469:errorcluster, "Value"=w466:variant)  [unwired: 1 out]
            n201 = Variant To Data(error in=w469, type=path "", Variant=w466) -> (data=w467:path, error out=w468:errorcluster)
            n202 = Bundle By Name(cluster=w471, "界面控件.当前选择路径"=w467) -> (w470:T7)
          }
          frame 3 {
            n203 = property class="Ctl"(reference=w473, error in=w481) -> (error out=w478:errorcluster, "Value"=w476:variant)  [unwired: 1 out]
            n204 = Variant To Data(error in=w478, type="", Variant=w476) -> (data=w474:string, error out=w477:errorcluster)
            n205 = Bundle By Name(cluster=w480, "界面控件.控件名称"=w474) -> (w479:T7)
          }
        }
        n206 = Build Array (concatenate)(w447) -> (w446:string[])
        n207 = Bundle By Name(cluster=w439, "Error"=w440) -> (w448:T7)
      }
      frame "UI :Resp - GetVICtrlName" {
        # "获取PathVI中选定条件的控件名称，并将名称存入表格文件中。当修改表格文件后可以将表格中修改的名称的控件进行替换名称或更新。"
        n208 = Unbundle By Name(w486) -> ("Error"=w487:errorcluster)
        n209 = Build Array (concatenate)(w484, string[] ["MV :Actn - GetVICotrlName", "MV :Actn - WriteCtrlNameToExcel"] ("数组")) -> (w483:string[])
        n210 = Bundle By Name(cluster=w486, "Error"=w487) -> (w485:T7)
      }
      frame "UI :Resp - ReOrigin" {
        n211 = Unbundle By Name(w495) -> ("DynamicThreadsPath.ReOriginVI"=w489:path, "Error"=w496:errorcluster)
        n212 = Strip Path(path=w489) -> (name=w490:string)  [unwired: 1 out]
        n213 = Bundle By Name(cluster=w495, "Thread to Operate.Invoke Property"=T9 {"open front panel? (T)"=TRUE, "Reentrant? (F)"=FALSE, "Insert to Subpanel?(F)"=FALSE, "time out(5s)"=5.0}, "Thread to Operate.Queue Info.Thread Q Name"=w490, "Thread to Operate.Thread VI Path"=w489, "Error"=w496) -> (w494:T7)
        n214 = Build Array (concatenate)(w493, string[] ["MV :TM - Load Dynamic VI"]) -> (w492:string[])
      }
      frame "UI :Resp - Load Dynamic VI" {
        n215 = Unbundle By Name(w504) -> ("Dynamic VI Path.Thread Path"=w498:path, "Error"=w505:errorcluster)
        n216 = Strip Path(path=w498) -> (name=w499:string)  [unwired: 1 out]
        n217 = Bundle By Name(cluster=w504, "Thread to Operate.Invoke Property"=T9 {"open front panel? (T)"=TRUE, "Reentrant? (F)"=FALSE, "Insert to Subpanel?(F)"=FALSE, "time out(5s)"=5.0}, "Thread to Operate.Queue Info.Thread Q Name"=w499, "Thread to Operate.Thread VI Path"=w498, "Error"=w505) -> (w503:T7)
        n218 = Build Array (concatenate)(w502, string[] ["MV :TM - Load Dynamic VI"]) -> (w501:string[])
      }
      frame "UI :Resp - Load Reentrant VI" {
        n219 = Unbundle By Name(w508) -> ("Reentrant VI Path.Reentrant VI Count"=w514:u32, "Reentrant VI Path.Reentrant Thread Path"=w515:path, "Error"=w516:errorcluster)
        n220 = Increment(x=w514) -> (x+1=w513:u32)
        n221 = Strip Path(path=w515) -> (name=w512:string)  [unwired: 1 out]
        n222 = Number To Decimal String(number=w513) -> (decimal integer string=w509:string)  [unwired: 1 in]
        n223 = Concatenate Strings(w512, "-" ("字符串"), w509) -> (w510:string)
        n224 = Bundle By Name(cluster=w508, "Thread to Operate.Invoke Property"=T9 {"open front panel? (T)"=TRUE, "Reentrant? (F)"=TRUE, "Insert to Subpanel?(F)"=FALSE, "time out(5s)"=5.0}, "Thread to Operate.Queue Info.Thread Q Name"=w510, "Reentrant VI Path.Reentrant VI Count"=w513, "Thread to Operate.Thread VI Path"=w515, "Error"=w516) -> (w507:T7)
        n225 = Build Array (concatenate)(w519, string[] ["MV :TM - Load Reentrant VI"]) -> (w518:string[])
      }
      frame "UI :Resp - Load Engine" {
        n226 = Unbundle By Name(w527) -> ("Engine Path.Engine Path"=w521:path, "Error"=w528:errorcluster)
        n227 = Strip Path(path=w521) -> (name=w522:string)  [unwired: 1 out]
        n228 = Bundle By Name(cluster=w527, "Thread to Operate.Invoke Property"=T9 {"open front panel? (T)"=TRUE, "Reentrant? (F)"=FALSE, "Insert to Subpanel?(F)"=FALSE, "time out(5s)"=5.0}, "Thread to Operate.Queue Info.Thread Q Name"=w522, "Thread to Operate.Thread VI Path"=w521, "Error"=w528) -> (w526:T7)
        n229 = Build Array (concatenate)(w525, string[] ["MV :TM - Load Engine"]) -> (w524:string[])
      }
      frame "UI :Resp - Close Dynamic VI" {
        n230 = Unbundle By Name(w535) -> ("Dynamic VI Path.Thread Path"=w530:path, "Error"=w536:errorcluster)
        n231 = Strip Path(path=w530) -> (name=w529:string)  [unwired: 1 out]
        n232 = Bundle By Name(cluster=w535, "Thread to Operate.Queue Info.Thread Q Name"=w529, "Error"=w536) -> (w534:T7)
        n233 = Build Array (concatenate)(w533, string[] ["MV :TM - Clean Dynamic Thread", "MV :TM - Shut Down Threads"] ("数组")) -> (w532:string[])
      }
      frame "UI :Resp - Close Engine" {
        n234 = Unbundle By Name(w543) -> ("Engine Path.Engine Path"=w538:path, "Error"=w544:errorcluster)
        n235 = Strip Path(path=w538) -> (name=w537:string)  [unwired: 1 out]
        n236 = Bundle By Name(cluster=w543, "Thread to Operate.Queue Info.Thread Q Name"=w537, "Error"=w544) -> (w542:T7)
        n237 = Build Array (concatenate)(w541, string[] ["MV :TM - Clean Dynamic Thread", "MV :TM - Shut Down Threads"] ("数组")) -> (w540:string[])
      }
      frame "UI :Resp - Exit Event" {
        n238 = Unbundle By Name(w549) -> ("Error"=w550:errorcluster)
        n239 = Build Array (concatenate)(w547, string[] ["MV :TM - Clean All Dynamic Thread", "MV :TM - Shut Down Threads", "MV :Core - Exit System"] ("数组")) -> (w546:string[])
        n240 = Bundle By Name(cluster=w549, "Error"=w550) -> (w548:T7)
      }
    }
    n241 = Unbundle By Name(w52) -> ("Exit"=w55:bool)
  }
  n242 = while {
    shift-right: [w552] -> w11
    shift-left: w7 -> [w553]
    stop <- w551 stop-if-true
    # "SW Architecture - Producer Loop - Respone The UI Events"
    n243 = event shown="[7] \"获取控件引用\": 值改变" {
      selector: _ -> [_ _ _ _ _ _ _ _ _ _ _ _ _ _ _]
      dyn-events: _ -> [_ _ _ _ _ _ _ _ _ _ _ _ _ _ _]
      timeout: 100 -> [_ _ _ _ _ _ _ _ _ _ _ _ _ _ _]
      tunnel: w553 -> [w557 w561 w568 w576 w583 w591 w610 w624 w632 w640 w650 w658 w666 w674 w682]
      tunnel: [w558 w562 w567 w575 w582 w590 w609 w623 w631 w639 w649 w657 w665 w673 w681] -> w552
      event Timeout {
        n244 = event-data() -> ()  [unwired: 1 in, 1 out]
        n245 = Unbundle By Name(w557) -> ("Main VI.Main Name"=w556:string)
        n246 = call <vilib>:"SA Verify Queue.vi"("Queue Name in"=w556) -> ("Not A Queue?"=w555:bool)  [unwired: 6 in, 3 out]
        n247 = Bundle By Name(cluster=w557, "Exit"=w555) -> (w558:T7)
      }
      event "创建数量": Value Change {
        n248 = event-data() -> ("NewVal"=w559:u16)  [unwired: 1 in]
        n249 = Unbundle By Name(w561) -> ("Error"=w560:errorcluster)
        n250 = Bundle By Name(cluster=w561, "控件排布前面板.创建控件.创建数量"=w559, "Error"=w560) -> (w562:T7)
      }
      event Panel Close? {
        n251 = event-data() -> ()  [unwired: 1 in, 1 out]
        n252 = Unbundle By Name(w568) -> ("Main VI.Main Name"=w564:string, "Error"=w569:errorcluster)
        n253 = call <vilib>:"SA Insert to Queue.vi"("error in"=w569, "Event"="UI :Resp - Exit Event", "Queue Name"=w564) -> ("error out"=w566:errorcluster)  [unwired: 8 in]
        n254 = Bundle By Name(cluster=w568, "Error"=w566) -> (w567:T7)
        n255 = event-data("Discard?"=TRUE ("放弃？")) -> ()  [unwired: 1 in, 1 out]
      }
      event "Exit Program", "停止": Value Change {
        n256 = event-data() -> ("CtlRef"=w572:refnum<vi>)  [unwired: 1 in]
        n257 = Unbundle By Name(w576) -> ("Main VI.Main Name"=w573:string, "Error"=w577:errorcluster)
        n258 = call <vilib>:"SA Insert to Queue.vi"("error in"=w577, "Event"="UI :Resp - Exit Event", "Queue Name"=w573) -> ("error out"=w571:errorcluster)  [unwired: 8 in]
        n259 = invoke class="Bool" method="Reinit To Default"(reference=w572, error in=w571) -> (error out=w570:errorcluster)  [unwired: 1 in, 2 out]
        n260 = Bundle By Name(cluster=w576, "Error"=w570) -> (w575:T7)
      }
      event "OK": Value Change {
        n261 = event-data() -> ("CtlRef"=w585:refnum<vi>)  [unwired: 1 in]
        n262 = Unbundle By Name(w583) -> ("Main VI.Main Name"=w578:string, "Error"=w579:errorcluster)
        n263 = call <vilib>:"SA Insert to Queue.vi"("error in"=w579, "Event"="UI :Resp - /* ADD NAME */", "Queue Name"=w578) -> ("error out"=w580:errorcluster)  [unwired: 8 in]
        n264 = invoke class="Bool" method="Reinit To Default"(reference=w585, error in=w580) -> (error out=w584:errorcluster)  [unwired: 1 in, 2 out]
        n265 = Bundle By Name(cluster=w583, "Error"=w584) -> (w582:T7)
      }
      event "获取控件名称": Value Change {
        n266 = event-data() -> ("CtlRef"=w593:refnum<vi>)  [unwired: 1 in]
        n267 = Unbundle By Name(w591) -> ("Main VI.Main Name"=w586:string, "Error"=w587:errorcluster)
        n268 = call <vilib>:"SA Insert to Queue.vi"("error in"=w587, "Event"="UI :Resp - GetVICtrlName", "Queue Name"=w586) -> ("error out"=w588:errorcluster)  [unwired: 8 in]
        n269 = invoke class="Bool (严格)" method="Reinit To Default"(reference=w593, error in=w588) -> (error out=w592:errorcluster)  [unwired: 1 in, 2 out]
        n270 = Bundle By Name(cluster=w591, "Error"=w592) -> (w590:T7)
      }
      event "界面控件": Value Change {
        n271 = event-data() -> ("CtlRef"=w611:refnum<vi>, "OldVal"=w606:T2, "NewVal"=w605:T2)  [unwired: 1 in]
        n272 = Not Equal?(x=w606, y=w605) -> (x != y?=w604:T12)
        n273 = Unbundle By Name(w610) -> ("Main VI.Main Name"=w607:string, "Error"=w595:errorcluster)
        n274 = Cluster To Array(cluster=w604) -> (array=w603:bool[])
        n275 = Search 1D Array(1D array=w603, element=TRUE ("元素")) -> (index of element=w598:i32)  [unwired: 1 in]
        n276 = property class="Clust (严格)"(reference=w611, error in=w595) -> (error out=w594:errorcluster, "Controls[]"=w601:refnum<vi>[])  [unwired: 1 out]
        n277 = Index Array(array=w601, index=w598) -> (element=w599:refnum<vi>)
        n278 = Equal?(x=w598, y=-1) -> (x = y?=w596:bool)
        n279 = Bundle(w599, "index of element"=w598) -> (w600:cluster{refnum<vi>, "index of element":i32})  [unwired: 1 in]
        n280 = case shown="假" w596 {
          tunnel: [w616 w618] -> w608
          tunnel: w594 -> [w615 w618]
          tunnel: w607 -> [w614 _]
          tunnel: w600 -> [w612 _]
          frame False {
            n281 = To Variant(anything=w612) -> (Variant=w613:variant)
            n282 = call <vilib>:"SA Insert to Queue.vi"("error in"=w615, "Data"=w613, "Event"="UI :Resp - PlanCtrlChange", "Queue Name"=w614) -> ("error out"=w616:errorcluster)  [unwired: 7 in]
          }
          frame True {
          }
        }
        n283 = Bundle By Name(cluster=w610, "Error"=w608) -> (w609:T7)
      }
      event "获取控件引用": Value Change {
        n284 = event-data() -> ("CtlRef"=w626:refnum<vi>)  [unwired: 1 in]
        n285 = Unbundle By Name(w624) -> ("Main VI.Main Name"=w619:string, "Error"=w620:errorcluster)
        n286 = call <vilib>:"SA Insert to Queue.vi"("error in"=w620, "Event"="MV :Actn - GetCotrlRef", "Queue Name"=w619) -> ("error out"=w621:errorcluster)  [unwired: 8 in]
        n287 = invoke class="Bool" method="Reinit To Default"(reference=w626, error in=w621) -> (error out=w625:errorcluster)  [unwired: 1 in, 2 out]
        n288 = Bundle By Name(cluster=w624, "Error"=w625) -> (w623:T7)
      }
      event "Load Engine VI": Value Change {
        n289 = event-data() -> ("CtlRef"=w634:refnum<vi>)  [unwired: 1 in]
        n290 = Unbundle By Name(w632) -> ("Main VI.Main Name"=w627:string, "Error"=w628:errorcluster)
        n291 = call <vilib>:"SA Insert to Queue.vi"("error in"=w628, "Event"="UI :Resp - Load Engine", "Queue Name"=w627) -> ("error out"=w629:errorcluster)  [unwired: 8 in]
        n292 = invoke class="Bool" method="Reinit To Default"(reference=w634, error in=w629) -> (error out=w633:errorcluster)  [unwired: 1 in, 2 out]
        n293 = Bundle By Name(cluster=w632, "Error"=w633) -> (w631:T7)
      }
      event "重定原点": Value Change {
        n294 = event-data() -> ("CtlRef"=w642:refnum<vi>)  [unwired: 1 in]
        n295 = Unbundle By Name(w640) -> ("Main VI.Main Name"=w635:string, "Error"=w636:errorcluster)
        n296 = call <vilib>:"SA Insert to Queue.vi"("error in"=w636, "Event"="UI :Resp - ReOrigin", "Queue Name"=w635) -> ("error out"=w637:errorcluster)  [unwired: 8 in]
        n297 = invoke class="Bool" method="Reinit To Default"(reference=w642, error in=w637) -> (error out=w641:errorcluster)  [unwired: 1 in, 2 out]
        n298 = Bundle By Name(cluster=w640, "Error"=w641) -> (w639:T7)
      }
      event "创建T控件": Value Change {
        n299 = event-data() -> ("CtlRef"=w652:refnum<vi>)  [unwired: 1 in]
        n300 = Unbundle By Name(w650) -> ("Main VI.Main Name"=w644:string, "Error"=w646:errorcluster)
        n301 = call <vilib>:"SA Insert to Queue.vi"("error in"=w646, "Event"="MV :Actn - GetCotrlNameLable", "Queue Name"=w644) -> ("error out"=w645:errorcluster)  [unwired: 8 in]
        n302 = call <vilib>:"SA Insert to Queue.vi"("error in"=w645, "Event"="MV :Actn - CreateCotrl", "Queue Name"=w644) -> ("error out"=w647:errorcluster)  [unwired: 8 in]
        n303 = invoke class="Bool" method="Reinit To Default"(reference=w652, error in=w647) -> (error out=w651:errorcluster)  [unwired: 1 in, 2 out]
        n304 = Bundle By Name(cluster=w650, "Error"=w651) -> (w649:T7)
      }
      event "Close Engine VI": Value Change {
        n305 = event-data() -> ("CtlRef"=w660:refnum<vi>)  [unwired: 1 in]
        n306 = Unbundle By Name(w658) -> ("Main VI.Main Name"=w653:string, "Error"=w654:errorcluster)
        n307 = call <vilib>:"SA Insert to Queue.vi"("error in"=w654, "Event"="UI :Resp - Close Engine", "Queue Name"=w653) -> ("error out"=w655:errorcluster)  [unwired: 8 in]
        n308 = invoke class="Bool" method="Reinit To Default"(reference=w660, error in=w655) -> (error out=w659:errorcluster)  [unwired: 1 in, 2 out]
        n309 = Bundle By Name(cluster=w658, "Error"=w659) -> (w657:T7)
      }
      event "Load Dynamic VI": Value Change {
        n310 = event-data() -> ("CtlRef"=w668:refnum<vi>)  [unwired: 1 in]
        n311 = Unbundle By Name(w666) -> ("Main VI.Main Name"=w661:string, "Error"=w663:errorcluster)
        n312 = call <vilib>:"SA Insert to Queue.vi"("error in"=w663, "Event"="UI :Resp - Load Dynamic VI", "Queue Name"=w661) -> ("error out"=w662:errorcluster)  [unwired: 8 in]
        n313 = invoke class="Bool" method="Reinit To Default"(reference=w668, error in=w662) -> (error out=w667:errorcluster)  [unwired: 1 in, 2 out]
        n314 = Bundle By Name(cluster=w666, "Error"=w667) -> (w665:T7)
      }
      event "Load Reentrant VI": Value Change {
        n315 = event-data() -> ("CtlRef"=w676:refnum<vi>)  [unwired: 1 in]
        n316 = Unbundle By Name(w674) -> ("Main VI.Main Name"=w669:string, "Error"=w671:errorcluster)
        n317 = call <vilib>:"SA Insert to Queue.vi"("error in"=w671, "Event"="UI :Resp - Load Reentrant VI", "Queue Name"=w669) -> ("error out"=w670:errorcluster)  [unwired: 8 in]
        n318 = invoke class="Bool" method="Reinit To Default"(reference=w676, error in=w670) -> (error out=w675:errorcluster)  [unwired: 1 in, 2 out]
        n319 = Bundle By Name(cluster=w674, "Error"=w675) -> (w673:T7)
      }
      event "Close Dynamic VI": Value Change {
        n320 = event-data() -> ("CtlRef"=w684:refnum<vi>)  [unwired: 1 in]
        n321 = Unbundle By Name(w682) -> ("Main VI.Main Name"=w677:string, "Error"=w678:errorcluster)
        n322 = call <vilib>:"SA Insert to Queue.vi"("error in"=w678, "Event"="UI :Resp - Close Dynamic VI", "Queue Name"=w677) -> ("error out"=w679:errorcluster)  [unwired: 8 in]
        n323 = invoke class="Bool" method="Reinit To Default"(reference=w684, error in=w679) -> (error out=w683:errorcluster)  [unwired: 1 in, 2 out]
        n324 = Bundle By Name(cluster=w682, "Error"=w683) -> (w681:T7)
      }
    }
    n325 = Unbundle By Name(w552) -> ("Exit"=w551:bool)
  }
  n326 = disable-structure shown="\"Event Source\"" {
    frame condition #0 (active) {
    }
    frame condition #1 {
    }
  }
  n327 = Unbundle By Name(w11) -> ("Error"=w12:errorcluster)
  n328 = call <vilib>:"SA Application Exit.vi"("error in"=w12) -> ()  [unwired: 10 in, 1 out]
  n329 = Unbundle By Name(w2) -> ("Main VI.Main Name"=w5:string, "Error"=w3:errorcluster)
  n330 = disable-structure shown="启用" {
    frame Disabled {
    }
    frame Enabled {
    }
  }
  n331 = disable-structure shown="禁用" {
    frame Disabled {
      (unwired) "MV :Actn - GetCotrlRef" ("Event")
      n332 = To Variant() -> ()  [unwired: 1 in, 1 out]
      n333 = Variant To Data() -> ()  [unwired: 3 in, 2 out]
    }
    frame Enabled {
    }
  }
  n334 = call <vilib>:"SA Destroy Queue.vi"("error in"=w3, "Queue Name"=w5) -> ()  [unwired: 9 in, 1 out]
